vi "Steuerprogramm02-15.vi"() -> ()   [LabVIEW 2010]
uses:
  <vilib>/rvi/interface/nirviReadWriteControl/nirviReadWriteControl.xnode
  <vilib>/rvi/errors/niLvFpgaWhatHappensToTopLevelVI.ctl
  <vilib>/rvi/interface/common/niFpgaNodeNameForErrorReporting.ctl
  <vilib>/rvi/errors/niLvFpgaAdjustHostInterfaceError.vi
  gvbooleschRT.vi
  <vilib>/functionblocks/FB Core/FB Core.xnode
  <vilib>/functionblocks/Counter/Elapsed Timer/Elapsed Timer.vi
  <vilib>/functionblocks/NI_FunctionBlock Libraries.lvlib
  <vilib>/rvi/interface/nirviCloseFPGA/nirviCloseFPGA.xnode
  <vilib>/addons/control/pid/NI_PID_pid.lvlib
  C:/Users/HAGAR-IV/Desktop/Zeugs/Johnny/pertrasgc fpga/FPGA-Programm-10-14.vi
  C:/Users/HAGAR-IV/Desktop/Zeugs/markus/version feb 2012/FPGA Bitfiles/pertrasgcfpga2_FPGATarget_FPGA-Programm-10_16368CB6.lvbitx
  NiFpgaLv.dll
  <vilib>/Utility/error.llb/Error Cluster From Error Code.vi
  GVMWHorst.vi
  GVMethodenwechsel.vi
  GVHorstSP.vi
  GVZwangs.vi
  GVHK1Hz.vi
  GVHeizenLH.vi
  GVAIs.vi
  <vilib>/addons/control/pid/pid.llb/PID (DBL Array).vi
  GVTrapsMachs.vi
  GVaktuelleTDMS.vi
  GVECDs.vi
  GVZeitenZyklen.vi
  GVProbenvol.vi
  GVVentilposition.vi
  <vilib>/FPGAPlugInAG/cRIO-9114/niLvFpga_Close_cRIO-9114.vi
panel:
  in  "Methode speichern":bool
  in  "DetYMax":dbl
  in  "DetYMin":dbl
  in  "HK2YMax":dbl
  in  "HK2YMin":dbl
  in  "HK1YMax":dbl
  in  "HK1YMin":dbl
  out "ZyklusNummernGesamt":i32[](array[numeric])
  in  "Detektor":i32(ring) items=["ECD1", "ECD2"]
  out "Detektor":cluster{dbl[], dbl[]}[](graph)
  out "Zykluslängen [s]":dbl[](array[numeric])
  in  "veränderte Methode benutzen":bool
  in  "Methode verändern":bool
  in  "dargestellte Größe 2":i32(ring)=1 items=["T-MainCol3", "T-Trap1", "T-Trap2", "T-Stirling", "T-PreCol1", "T-PreCol2", "T-MainCol1", "T-MainCol2", "T-T-Line2", "T-MI1", "T-MI2", "T-MI3", "T-MI4", "T-MI5", "T-MI6", "F-MFM1", "T-MainCol4", "T-BHorst1", "T-BHorst2", "T-BHorst3", "T-BHorst4", "T-Oven1", "T-Oven2", "T-T-Line1", "F-MFM2", "P-Me-HP", "P-Me-LP", "P-Vac", "Ref-Turbo", "I-MS-AC", "I-Trap1", "I-Trap2", "Mod2/AI0", "Mod2/AI1", "Mod2/AI2", "Mod2/AI3", "Mod2/AI4", "Mod2/AI5", "Mod2/AI6", "Mod2/AI7", "Mod2/AI8", "Mod2/AI9", "Mod2/AI10", "Mod2/AI11", "Mod2/AI12", "Mod2/AI13", "Mod2/AI14", "Mod2/AI15", "Mod2/AI16", "Mod2/AI17", "Mod2/AI18", "Mod2/AI19", "Mod2/AI20", "Mod2/AI21", "Mod2/AI22", "Mod2/AI23", "Mod2/AI24", "Mod2/AI25", "Mod2/AI26", "Mod2/AI27", "Mod2/AI28", "Mod2/AI29", "Mod2/AI30", "Mod2/AI31", "Mod3/AI0", "Mod3/AI1", "Mod3/AI2", "Mod3/AI3", "Mod3/AI4", "Mod3/AI5", "Mod3/AI6", "Mod3/AI7", "Mod3/AI8", "Mod3/AI9", "Mod3/AI10", "Mod3/AI11", "Mod3/AI12", "Mod3/AI13", "Mod3/AI14", "Mod3/AI15", "Mod3/AI16", "Mod3/AI17", "Mod3/AI18", "Mod3/AI19", "Mod3/AI20", "Mod3/AI21", "Mod3/AI22", "Mod3/AI23", "Mod3/AI24", "Mod3/AI25", "Mod3/AI26", "Mod3/AI27", "Mod3/AI28", "Mod3/AI29", "Mod3/AI30", "Mod3/AI31", "U_Widr.Trap1 [V]", "Temp.Trap1 [°C]", "U_Widr.Trap2 [V]", "Temp.Trap2 [°C]", "Temp.Mach1 [°C]", "Temp.Mach2 [°C]", "MFC1B", "PressContr1A", "PressContr1B", "PressContr1C", "MFC1A", "PressContr1D", "MFC1A Integriert"]
  in  "Zeitachse2":i32(ring)=1 items=["Zykluszeit [s] Mod0", "Zykluszeit [s] Mod1", "Zykluszeit [s] Mod2A", "Zykluszeit [s] Mod2B"]
  out "Housekeeping2":cluster{dbl[], dbl[]}(graph)
  out "ZyklusNummern":i32[](array[numeric])
  in  "dargestellte Größe 1":i32(ring)=1 items=["T-MainCol3", "T-Trap1", "T-Trap2", "T-Stirling", "T-PreCol1", "T-PreCol2", "T-MainCol1", "T-MainCol2", "T-T-Line2", "T-MI1", "T-MI2", "T-MI3", "T-MI4", "T-MI5", "T-MI6", "F-MFM1", "T-MainCol4", "T-BHorst1", "T-BHorst2", "T-BHorst3", "T-BHorst4", "T-Oven1", "T-Oven2", "T-T-Line1", "F-MFM2", "P-Me-HP", "P-Me-LP", "P-Vac", "Ref-Turbo", "I-MS-AC", "I-Trap1", "I-Trap2", "Mod2/AI0", "Mod2/AI1", "Mod2/AI2", "Mod2/AI3", "Mod2/AI4", "Mod2/AI5", "Mod2/AI6", "Mod2/AI7", "Mod2/AI8", "Mod2/AI9", "Mod2/AI10", "Mod2/AI11", "Mod2/AI12", "Mod2/AI13", "Mod2/AI14", "Mod2/AI15", "Mod2/AI16", "Mod2/AI17", "Mod2/AI18", "Mod2/AI19", "Mod2/AI20", "Mod2/AI21", "Mod2/AI22", "Mod2/AI23", "Mod2/AI24", "Mod2/AI25", "Mod2/AI26", "Mod2/AI27", "Mod2/AI28", "Mod2/AI29", "Mod2/AI30", "Mod2/AI31", "Mod3/AI0", "Mod3/AI1", "Mod3/AI2", "Mod3/AI3", "Mod3/AI4", "Mod3/AI5", "Mod3/AI6", "Mod3/AI7", "Mod3/AI8", "Mod3/AI9", "Mod3/AI10", "Mod3/AI11", "Mod3/AI12", "Mod3/AI13", "Mod3/AI14", "Mod3/AI15", "Mod3/AI16", "Mod3/AI17", "Mod3/AI18", "Mod3/AI19", "Mod3/AI20", "Mod3/AI21", "Mod3/AI22", "Mod3/AI23", "Mod3/AI24", "Mod3/AI25", "Mod3/AI26", "Mod3/AI27", "Mod3/AI28", "Mod3/AI29", "Mod3/AI30", "Mod3/AI31", "U_Widr.Trap1 [V]", "Temp.Trap1 [°C]", "U_Widr.Trap2 [V]", "Temp.Trap2 [°C]", "Temp.Mach1 [°C]", "Temp.Mach2 [°C]", "MFC1B", "PressContr1A", "PressContr1B", "PressContr1C", "MFC1A", "PressContr1D", "MFC1A Integriert"]
  in  "Zeitachse1":i32(ring)=1 items=["Zykluszeit [s] Mod0", "Zykluszeit [s] Mod1", "Zykluszeit [s] Mod2A", "Zykluszeit [s] Mod2B"]
  out "Housekeeping1":cluster{dbl[], dbl[]}(graph)
  out "Big Ben, Methodenzeit, Zykluszeit0, Zykluszeit1, Zykluszeit2A, Zykluszeit2B":dbl[](array[numeric])
  in  "global stop RT":bool
  in  "Methode":i32(ring) items=["0"]
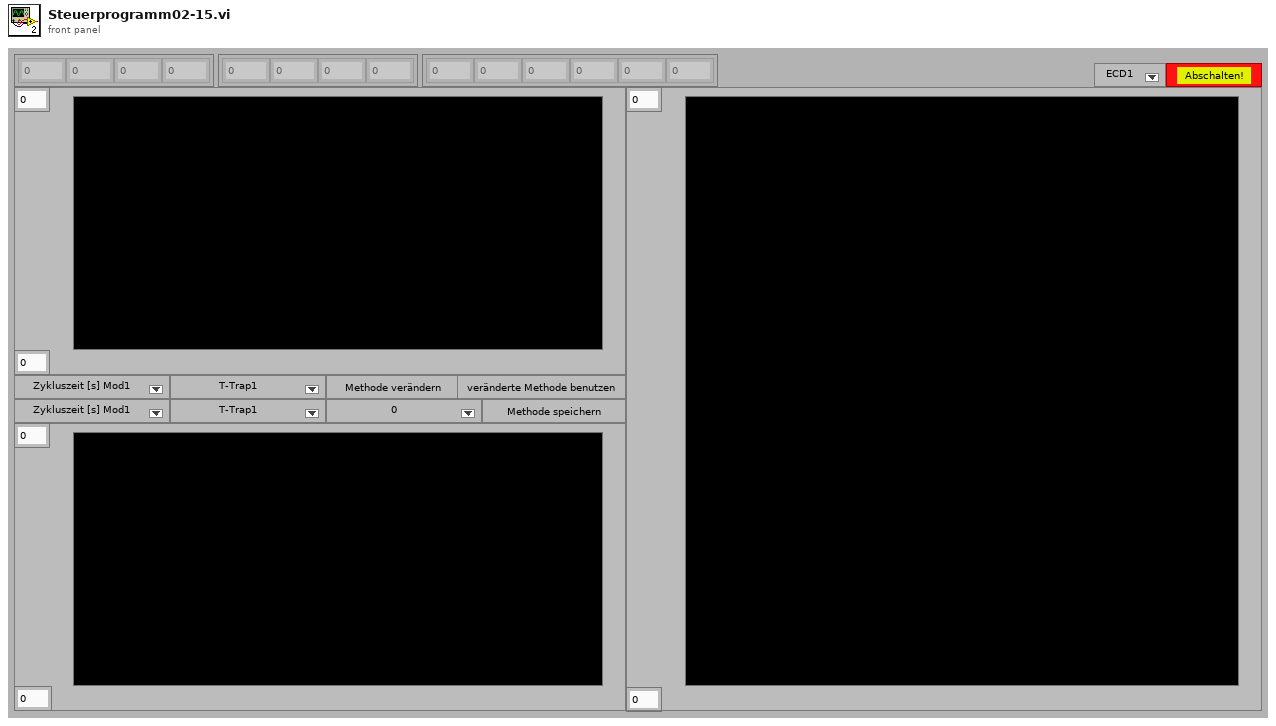
[diagram p1: front panel]
types:
  T1 = cluster{"Zykluslängen [s]":dbl[], "ZeitpktDIOsMod0":dbl[], "ZeitpktDIOsMod1":dbl[], "ZeitpktDIOsMod2A":dbl[], "ZeitpktDIOsMod2B":dbl[], "DIOsSPMod0":bool[][], "DIOsSPMod1":bool[][], "DIOsSPMod2A":bool[][], "DIOsSPMod2B":bool[][], "Mod0HorstZeitpkt":dbl[], "Mod1HorstZeitpkt":dbl[], "Mod2AHorstZeitpkt":dbl[], "Mod2BHorstZeitpkt":dbl[], "HorstSPMod0":dbl[][], "HorstSPMod1":dbl[][], "HorstSPMod2A":dbl[][], "HorstSPMod2B":dbl[][], "LangsameHeizungenSP":dbl[], "LHHeizen?":bool[], "ZPktFPGABoolesch":dbl[], "FPGABoolesch":bool[][], "ZeitpktFPGAPID":dbl[], "FPGAPID":cluster{"proportional gain (Kc)":fxp<+/-,16,8>, "integral gain (Kc*Ts/Ti)":fxp<+/-,16,8>, "derivative gain (Kc*Td/Ts)":fxp<+/-,16,8>}[][], "ZeitpktFPGAFixp":dbl[], "FPGAFixp":fxp<+/-,16,4>[][], "ZeitpktMach1":dbl[], "TempMach1":dbl[], "ZeitpktMach2":dbl[], "TempMach2":dbl[], "PIDs für \"träge\" Heizungen":cluster{"proportional gain (Kc)":dbl, "integral time (Ti, min)":dbl, "derivative time (Td, min)":dbl}[], "Zwangsbedingungen":dbl[][], "Dateien fürs MS schicken?":bool, "ZeitpunkteMPV":dbl[], "SPMPV":i32[], "ZeitpktMSa":dbl, "ZeitpktMSb":dbl, "Int.Start1":dbl, "Int.Stop1":dbl, "Int.Start2":dbl, "Int.Stop2":dbl, "Methodenname":string}[]
  T2 = cluster{"DIOsMod0Nr":i32[], "DIOsMod1Nr":i32[], "DIOsMod2ANr":i32[], "DIOsMod2BNr":i32[], "AIsLH":i32[], "Anzahl Horst/Modul":i32[], "Regler für den Probenfluß":i32, "StringSPvorgebenMod0":string[], "StringSPvorgebenMod1":string[], "StringSPvorgebenMod2A":string[], "StringSPvorgebenMod2B":string[], "StringMWAntwort0":string[], "StringMWAntwort1":string[], "StringMWAntwort2A":string[], "StringMWAntwort2B":string[], "UmrechnungHorst0":dbl[], "UmrechnungHorst1":dbl[], "UmrechnungHorst2A":dbl[], "UmrechnungHorst2B":dbl[], "StringMWabfragenMod0":string[], "StringMWabfragenMod1":string[], "StringMWabfragenMod2A":string[], "StringMWabfragenMod2B":string[], "Modul1/AI koeff":dbl[][], "Modul2/AI koeff":dbl[][], "Modul3/AI koeff":dbl[][], "Traps/MachsKoeff":dbl[][], "Modul1/AIsNamen":string[], "Modul2/AIsNamen":string[], "Modul3/AIsNamen":string[], "DIOsMod0Name":string[], "DIOsMod1Name":string[], "DIOsMod2AName":string[], "DIOsMod2BName":string[], "HorstMod0Name":string[], "HorstMod1Name":string[], "HorstMod2AName":string[], "HorstMod2BName":string[], "Startmethode":i32, "Dateiordner Housekeeping":path, "Dateiname Housekeeping":string, "DateiordnerECD1":path, "DateinameECD1":string, "DateiordnerECD2":path, "DateinameECD2":string, "NamenLangsameHeizungen":string[], "ModuleLH":i32[]}
  T3 = enum16{"open", "replace", "create", "open or create", "replace or create", "replace or create with confirmation"}
  T4 = cluster{"DIOsMod0Nr":i32[], "DIOsMod1Nr":i32[], "DIOsMod2ANr":i32[], "DIOsMod2BNr":i32[], "AIs für \"träge\" Heizungen":i32[], i32[], "AnschlüsseHorstMod0":enum8{"0", "1", "2", "3", "4", "5", "6", "7", "8"}[], "AnschlüsseHorstMod1":enum8{"0", "1", "2", "3", "4", "5", "6", "7", "8"}[], "AnschlüsseHorstMod2A":enum8{"0", "1", "2", "3", "4", "5", "6", "7", "8"}[], "AnschlüsseHorstMod2B":enum8{"0", "1", "2", "3", "4", "5", "6", "7", "8"}[], "StringSPvorgebenMod0":string[], "StringSPvorgebenMod1":string[], "StringSPvorgebenMod2A":string[], "StringSPvorgebenMod2B":string[], "StringMWAntwort0":string[], "StringMWAntwort1":string[], "StringMWAntwort2A":string[], "StringMWAntwort2B":string[], "UmrechnungHorst0":dbl[], "UmrechnungHorst1":dbl[], "UmrechnungHorst2A":dbl[], "UmrechnungHorst2B":dbl[], "StringMWabfragenMod0":string[], "StringMWabfragenMod1":string[], "StringMWabfragenMod2A":string[], "StringMWabfragenMod2B":string[], "Modul1/AI koeff":dbl[][], "Modul2/AI koeff":dbl[][], "Modul3/AI koeff":dbl[][], "Traps/MachKoeff":dbl[][], "AIsNamen":string[], "DIOsMod0Name":string[], "DIOsMod1Name":string[], "DIOsMod2AName":string[], "DIOsMod2BName":string[], "HorstMod0Name":string[], "HorstMod1Name":string[], "HorstMod2AName":string[], "HorstMod2BName":string[], "Startmethode":i32, "Dateiordner Housekeeping":path, "Dateiname Housekeeping":string, "DateiordnerECD1":path, "DateinameECD1":string, "DateiordnerECD2":path, "DateinameECD2":string}
  T5 = cluster{"Zykluslängen [s]":dbl[], "ZeitpktDIOsMod0":dbl[], "ZeitpktDIOsMod1":dbl[], "ZeitpktDIOsMod2A":dbl[], "ZeitpktDIOsMod2B":dbl[], "DIOsSPMod0":bool[][], "DIOsSPMod1":bool[][], "DIOsSPMod2A":bool[][], "DIOsSPMod2B":bool[][], "Mod0HorstZeitpkt":dbl[], "Mod1HorstZeitpkt":dbl[], "Mod2AHorstZeitpkt":dbl[], "Mod2BHorstZeitpkt":dbl[], "HorstSPMod0":dbl[][], "HorstSPMod1":dbl[][], "HorstSPMod2A":dbl[][], "HorstSPMod2B":dbl[][], "LangsameHeizungenSP":dbl[], "LHHeizen?":bool[], "ZPktFPGABoolesch":dbl[], "FPGABoolesch":bool[][], "ZeitpktFPGAPID":dbl[], "FPGAPID":cluster{"proportional gain (Kc)":fxp<+/-,16,8>, "integral gain (Kc*Ts/Ti)":fxp<+/-,16,8>, "derivative gain (Kc*Td/Ts)":fxp<+/-,16,8>}[][], "ZeitpktFPGAFixp":dbl[], "FPGAFixp":fxp<+/-,16,4>[][], "ZeitpktMach1":dbl[], "TempMach1":dbl[], "ZeitpktMach2":dbl[], "TempMach2":dbl[], "PIDs für \"träge\" Heizungen":cluster{"proportional gain (Kc)":dbl, "integral time (Ti, min)":dbl, "derivative time (Td, min)":dbl}[], "Zwangsbedingungen":dbl[][], "Text0 MS-Datei":string, "Info":string, "wie wird gespeichert?":u16, "Speicherlänge":string, "Dateien fürs MS schicken?":bool, "Pfad MS-Datei CRIO":path}[]
  T6 = cluster{"DIOsMod0Nr":i32[], "DIOsMod1Nr":i32[], "DIOsMod2ANr":i32[], "DIOsMod2BNr":i32[], "AIs für \"träge\" Heizungen":i32[], i32[], "AnschlüsseHorstMod0":enum8{"0", "1", "2", "3", "4", "5", "6", "7", "8"}[], "AnschlüsseHorstMod1":enum8{"0", "1", "2", "3", "4", "5", "6", "7", "8"}[], "AnschlüsseHorstMod2A":enum8{"0", "1", "2", "3", "4", "5", "6", "7", "8"}[], "AnschlüsseHorstMod2B":enum8{"0", "1", "2", "3", "4", "5", "6", "7", "8"}[], "StringSPvorgebenMod0":string[], "StringSPvorgebenMod1":string[], "StringSPvorgebenMod2A":string[], "StringSPvorgebenMod2B":string[], "StringMWAntwort0":string[], "StringMWAntwort1":string[], "StringMWAntwort2A":string[], "StringMWAntwort2B":string[], "UmrechnungHorst0":dbl[], "UmrechnungHorst1":dbl[], "UmrechnungHorst2A":dbl[], "UmrechnungHorst2B":dbl[], "StringMWabfragenMod0":string[], "StringMWabfragenMod1":string[], "StringMWabfragenMod2A":string[], "StringMWabfragenMod2B":string[], "Modul1/AI koeff":dbl[][], "Modul2/AI koeff":dbl[][], "Modul3/AI koeff":dbl[][], "Traps/MachKoeff":dbl[][], "AIsNamen":string[], "DIOsMod0Name":string[], "DIOsMod1Name":string[], "DIOsMod2AName":string[], "DIOsMod2BName":string[], "HorstMod0Name":string[], "HorstMod1Name":string[], "HorstMod2AName":string[], "HorstMod2BName":string[], "Startmethode":i32, "Dateiordner Housekeeping":path, "Dateiname Housekeeping":string}
  T7 = cluster{"Zyklus1":i32, "Zeitachse1":i32, "dargestellte Größe 1":i32, "Zyklus2":i32, "Zeitachse2":i32, "dargestellte Größe 2":i32}
  T8 = typedef "niFpgaNodeNameForErrorReporting.ctl" = enum16{"Open FPGA VI Reference", "Read/Write Control", "Invoke Method: Abort", "Invoke Method: Acknowledge IRQ", "Invoke Method: Download", "Invoke Method: FIFO.Configure", "Invoke Method: FIFO.Read", "Invoke Method: FIFO.Start", "Invoke Method: FIFO.Stop", "Invoke Method: FIFO.Write", "Invoke Method: Reset", "Invoke Method: Run", "Invoke Method: Wait on IRQ", "Close FPGA VI Reference"}
  T9 = typedef "niLvFpgaWhatHappensToTopLevelVI.ctl" = enum16{"top level VI scripted behind XNode", "top level VI inlined behind XNode"}
  T10 = cluster{"DIOsMod0Name":string[], "DIOsMod1Name":string[], "DIOsMod2AName":string[], "DIOsMod2BName":string[], "HorstMod0Name":string[], "HorstMod1Name":string[], "HorstMod2AName":string[], "HorstMod2BName":string[], "NamenLangsameHeizungen":string[]}
  T11 = cluster{"Dateiordner Housekeeping":path, "DateiordnerECD1":path, "DateiordnerECD2":path, "Dateiname Housekeeping":string, "DateinameECD1":string, "DateinameECD2":string, "tdms0":refnum<k34>, "tdms1":refnum<k34>, "tdms0":refnum<k34>, "tdms1":refnum<k34>, "tdms0":refnum<k34>, "tdms1":refnum<k34>}
  T12 = cluster{"Zykluslängen [s]":dbl[], "ZeitpktDIOsMod0":dbl[], "ZeitpktDIOsMod1":dbl[], "ZeitpktDIOsMod2A":dbl[], "ZeitpktDIOsMod2B":dbl[], "DIOsSPMod0":bool[][], "DIOsSPMod1":bool[][], "DIOsSPMod2A":bool[][], "DIOsSPMod2B":bool[][], "Mod0HorstZeitpkt":dbl[], "Mod1HorstZeitpkt":dbl[], "Mod2AHorstZeitpkt":dbl[], "Mod2BHorstZeitpkt":dbl[], "HorstSPMod0":dbl[][], "HorstSPMod1":dbl[][], "HorstSPMod2A":dbl[][], "HorstSPMod2B":dbl[][], "LangsameHeizungenSP":dbl[], "LHHeizen?":bool[], "ZPktFPGABoolesch":dbl[], "FPGABoolesch":bool[][], "ZeitpktFPGAPID":dbl[], "FPGAPID":cluster{"proportional gain (Kc)":fxp<+/-,16,8>, "integral gain (Kc*Ts/Ti)":fxp<+/-,16,8>, "derivative gain (Kc*Td/Ts)":fxp<+/-,16,8>}[][], "ZeitpktFPGAFixp":dbl[], "FPGAFixp":fxp<+/-,16,4>[][], "ZeitpktMach1":dbl[], "TempMach1":dbl[], "ZeitpktMach2":dbl[], "TempMach2":dbl[], "PIDs für \"träge\" Heizungen":cluster{"proportional gain (Kc)":dbl, "integral time (Ti, min)":dbl, "derivative time (Td, min)":dbl}[], "Zwangsbedingungen":dbl[][], "Dateien fürs MS schicken?":bool, "ZeitpunkteMPV":dbl[], "SPMPV":i32[], "ZeitpktMSa":dbl, "ZeitpktMSb":dbl, "Int.Start1":dbl, "Int.Stop1":dbl, "Int.Start2":dbl, "Int.Stop2":dbl, "Methodenname":string}
  T13 = cluster{"proportional gain (Kc)":fxp<+/-,16,8>, "integral gain (Kc*Ts/Ti)":fxp<+/-,16,8>, "derivative gain (Kc*Td/Ts)":fxp<+/-,16,8>}[][]
  T14 = cluster{"proportional gain (Kc)":dbl, "integral time (Ti, min)":dbl, "derivative time (Td, min)":dbl}[]
  T15 = cluster{"Heizen?LH[0]":bool, "Heizen?LH[1]":bool, "Heizen?LH[2]":bool, "Heizen?LH[3]":bool, "Heizen?LH[4]":bool, "Heizen?LH[5]":bool}
  T16 = cluster{"[0]":u32, "[1]":u32, "[2]":u32, "[3]":u32, "[4]":u32, "[5]":u32}
  T17 = cluster{cluster{"ZeitpktDIOsMod2B":dbl[]}[], cluster{"DIOsSPMod2B":bool[][]}[], cluster{"Mod2BHorstZeitpkt":dbl[]}[], cluster{"HorstSPMod2B":dbl[][]}[], "LHHeizen?":bool[], "ZPktFPGABoolesch":dbl[], "FPGABoolesch":bool[][], "ZeitpktFPGAPID":dbl[], "FPGAPID":cluster{"proportional gain (Kc)":fxp<+/-,16,8>, "integral gain (Kc*Ts/Ti)":fxp<+/-,16,8>, "derivative gain (Kc*Td/Ts)":fxp<+/-,16,8>}[][], "ZeitpktFPGAFixp":dbl[], "FPGAFixp":fxp<+/-,16,4>[][], "ZeitpktMach1":dbl[], "TempMach1":dbl[], "ZeitpktMach2":dbl[], "TempMach2":dbl[], "ZeitpunkteMPV":dbl[], "SPMPV":i32[]}
  T18 = cluster{"ZyklusNummern":i32[], "ZeilennummernDIOs":i32[], "ZwangsDIO?":cluster{bool[]}[], "ZeilennummernHorst":i32[], "ZwangsHorst?":cluster{bool[]}[], "ZeileFPGABoolesch":i32, "ZwangsFPGABoolesch?":bool[], "ZeileFPGAPID":i32, "ZeileFPGAFixp":i32, "ZeileMach1":i32, "ZeileMach2":i32, "ZeilennummerMPV":i32}
  T19 = cluster{"Zyklusnummern 0, 1, 2A, 2B":i32[], i32[], "ZwangsDIO?":cluster{bool[]}[], i32[], "ZwangsHorst?":cluster{bool[]}[], i32, "ZwangsFPGABoolesch?":bool[], i32, i32, i32, i32, "ZeilennummerMPV":i32}
  T20 = cluster{string[], string[], string[], dbl[], dbl[], dbl[]}
  T21 = cluster{string[], string[], string[], string, string}
  T22 = cluster{"Befehle1":string[], "Befehle2":string[], "Befehle3":string[]}
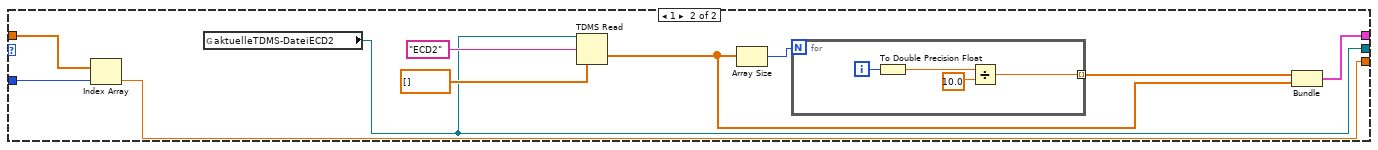
[diagram p6: hidden frame]
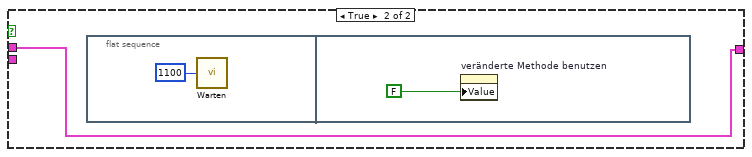
[diagram p7: hidden frame]
diagram:
  (unwired) T4 {"DIOsMod0Nr"=[], "DIOsMod1Nr"=[], "DIOsMod2ANr"=[], "DIOsMod2BNr"=[], "AIs für \"träge\" Heizungen"=[], [], "AnschlüsseHorstMod0"=[], "AnschlüsseHorstMod1"=[], "AnschlüsseHorstMod2A"=[], "AnschlüsseHorstMod2B"=[], "StringSPvorgebenMod0"=[], "StringSPvorgebenMod1"=[], "StringSPvorgebenMod2A"=[], "StringSPvorgebenMod2B"=[], "StringMWAntwort0"=[], "StringMWAntwort1"=[], "StringMWAntwort2A"=[], "StringMWAntwort2B"=[], "UmrechnungHorst0"=[], "UmrechnungHorst1"=[], "UmrechnungHorst2A"=[], "UmrechnungHorst2B"=[], "StringMWabfragenMod0"=[], "StringMWabfragenMod1"=[], "StringMWabfragenMod2A"=[], "StringMWabfragenMod2B"=[], "Modul1/AI koeff"=[], "Modul2/AI koeff"=[], "Modul3/AI koeff"=[], "Traps/MachKoeff"=[], "AIsNamen"=[], "DIOsMod0Name"=[], "DIOsMod1Name"=[], "DIOsMod2AName"=[], "DIOsMod2BName"=[], "HorstMod0Name"=[], "HorstMod1Name"=[], "HorstMod2AName"=[], "HorstMod2BName"=[], "Startmethode"=0, "Dateiordner Housekeeping"=path "", "Dateiname Housekeeping"="", "DateiordnerECD1"=path "", "DateinameECD1"="", "DateiordnerECD2"=path "", "DateinameECD2"=""} ("Einstellungen")
  (unwired) T5 [{"Zykluslängen [s]"=[180.0, 180.0, 180.0, 180.0], "ZeitpktDIOsMod0"=[0.0, 180.0], "ZeitpktDIOsMod1"=[0.0, 2.0, 15.0, 60.0, 61.0, 70.0, 80.0, 170.0, 180.0], "ZeitpktDIOsMod2A"=[0.0, 180.0], "ZeitpktDIOsMod2B"=[0.0, 60.0, 180.0], "DIOsSPMod0"=[[FALSE], [FALSE]], "DIOsSPMod1"=[[TRUE, TRUE, FALSE, TRUE, FALSE, TRUE, TRUE, TRUE, FALSE, FALSE, TRUE, FALSE, FALSE, FALSE, FALSE, FALSE, FALSE, TRUE], [TRUE, FALSE, FALSE, TRUE, FALSE, TRUE, TRUE, TRUE, FALSE, FALSE, TRUE, FALSE, FALSE, FALSE, FALSE, FALSE, FALSE, TRUE], [TRUE, FALSE, FALSE, FALSE, FALSE, TRUE, TRUE, FALSE, FALSE, FALSE, TRUE, FALSE, FALSE, FALSE, FALSE, FALSE, TRUE, TRUE], [TRUE, FALSE, FALSE, FALSE, FALSE, FALSE, TRUE, FALSE, FALSE, FALSE, TRUE, FALSE, FALSE, FALSE, FALSE, FALSE, TRUE, TRUE], [TRUE, FALSE, FALSE, FALSE, FALSE, FALSE, TRUE, FALSE, FALSE, FALSE, TRUE, FALSE, FALSE, FALSE, FALSE, FALSE, TRUE, TRUE], [TRUE, FALSE, FALSE, FALSE, FALSE, FALSE, TRUE, FALSE, FALSE, FALSE, TRUE, FALSE, FALSE, FALSE, FALSE, FALSE, TRUE, TRUE], [TRUE, FALSE, FALSE, FALSE, FALSE, FALSE, TRUE, FALSE, FALSE, FALSE, TRUE, FALSE, FALSE, FALSE, FALSE, FALSE, FALSE, TRUE], [TRUE, FALSE, FALSE, FALSE, FALSE, FALSE, TRUE, FALSE, FALSE, FALSE, TRUE, FALSE, FALSE, FALSE, FALSE, FALSE, FALSE, TRUE], [TRUE, FALSE, FALSE, FALSE, FALSE, FALSE, TRUE, FALSE, FALSE, FALSE, TRUE, FALSE, FALSE, FALSE, FALSE, FALSE, FALSE, TRUE]], "DIOsSPMod2A"=[[FALSE], [FALSE]], "DIOsSPMod2B"=[[FALSE], [FALSE]], "Mod0HorstZeitpkt"=[0.0, 180.0], "Mod1HorstZeitpkt"=[0.0, 55.0, 75.0, 180.0], "Mod2AHorstZeitpkt"=[0.0, 20.0, 180.0], "Mod2BHorstZeitpkt"=[0.0, 380.0], "HorstSPMod0"=[[2.66], [2.66]], "HorstSPMod1"=[[1.9, 0.0, 1.2], [0.0, 0.0, 1.2], [1.9, 0.0, 1.2], [1.9, 0.0, 1.2]], "HorstSPMod2A"=[[300.0], [300.0], [300.0]], "HorstSPMod2B"=[[0.0], [0.0]], "LangsameHeizungenSP"=[60.0, 220.0, 120.0, 60.0, 110.0, 0.0], "LHHeizen?"=[FALSE, TRUE, TRUE, FALSE, TRUE, FALSE], "ZPktFPGABoolesch"=[0.0, 60.0, 75.0, 180.0], "FPGABoolesch"=[[FALSE, FALSE, FALSE, FALSE, TRUE, FALSE], [FALSE, FALSE, TRUE, FALSE, TRUE, FALSE], [FALSE, FALSE, FALSE, FALSE, TRUE, FALSE], [FALSE, FALSE, FALSE, FALSE, TRUE, FALSE]], "ZeitpktFPGAPID"=[0.0, 60.0, 180.0], "FPGAPID"=[[{"proportional gain (Kc)"=5.0, "integral gain (Kc*Ts/Ti)"=0.0, "derivative gain (Kc*Td/Ts)"=0.0}, {"proportional gain (Kc)"=1.0, "integral gain (Kc*Ts/Ti)"=1.66796875, "derivative gain (Kc*Td/Ts)"=0.0}, {"proportional gain (Kc)"=5.0, "integral gain (Kc*Ts/Ti)"=0.03515625, "derivative gain (Kc*Td/Ts)"=0.0234375}, {"proportional gain (Kc)"=1.0, "integral gain (Kc*Ts/Ti)"=1.66796875, "derivative gain (Kc*Td/Ts)"=0.0}], [{"proportional gain (Kc)"=5.0, "integral gain (Kc*Ts/Ti)"=0.0, "derivative gain (Kc*Td/Ts)"=0.0}, {"proportional gain (Kc)"=1.0, "integral gain (Kc*Ts/Ti)"=1.66796875, "derivative gain (Kc*Td/Ts)"=0.0}, {"proportional gain (Kc)"=5.0, "integral gain (Kc*Ts/Ti)"=0.03515625, "derivative gain (Kc*Td/Ts)"=0.0234375}, {"proportional gain (Kc)"=1.0, "integral gain (Kc*Ts/Ti)"=1.66796875, "derivative gain (Kc*Td/Ts)"=0.0}], [{"proportional gain (Kc)"=0.0, "integral gain (Kc*Ts/Ti)"=0.0, "derivative gain (Kc*Td/Ts)"=0.0}, {"proportional gain (Kc)"=0.0, "integral gain (Kc*Ts/Ti)"=0.0, "derivative gain (Kc*Td/Ts)"=0.0}, {"proportional gain (Kc)"=2.0, "integral gain (Kc*Ts/Ti)"=0.03125, "derivative gain (Kc*Td/Ts)"=0.01953125}, {"proportional gain (Kc)"=0.0, "integral gain (Kc*Ts/Ti)"=0.0, "derivative gain (Kc*Td/Ts)"=0.0}], [{"proportional gain (Kc)"=0.0, "integral gain (Kc*Ts/Ti)"=0.0, "derivative gain (Kc*Td/Ts)"=0.0}, {"proportional gain (Kc)"=0.0, "integral gain (Kc*Ts/Ti)"=0.0, "derivative gain (Kc*Td/Ts)"=0.0}, {"proportional gain (Kc)"=2.0, "integral gain (Kc*Ts/Ti)"=0.03125, "derivative gain (Kc*Td/Ts)"=0.01953125}, {"proportional gain (Kc)"=0.0, "integral gain (Kc*Ts/Ti)"=0.0, "derivative gain (Kc*Td/Ts)"=0.0}], [{"proportional gain (Kc)"=0.0, "integral gain (Kc*Ts/Ti)"=0.0, "derivative gain (Kc*Td/Ts)"=0.0}, {"proportional gain (Kc)"=0.0, "integral gain (Kc*Ts/Ti)"=0.0, "derivative gain (Kc*Td/Ts)"=0.0}, {"proportional gain (Kc)"=2.0, "integral gain (Kc*Ts/Ti)"=0.03125, "derivative gain (Kc*Td/Ts)"=0.01953125}, {"proportional gain (Kc)"=0.0, "integral gain (Kc*Ts/Ti)"=0.0, "derivative gain (Kc*Td/Ts)"=0.0}]], "ZeitpktFPGAFixp"=[0.0, 60.0, 75.0, 180.0], "FPGAFixp"=[[0.0, 0.0, 0.0, 0.0, 0.0, 0.0, 2.85009765625, 0.0], [4.59423828125, 4.599365234375, 1.699951171875, 0.0, 0.0, 0.0, 2.85009765625, 0.0], [0.0, 0.0, 0.0, 0.0, 0.0, 0.0, 2.85009765625, 0.0], [0.0, 0.0, 0.0, 0.0, 0.0, 0.0, 2.85009765625, 0.0]], "ZeitpktMach1"=[0.0, 1.0, 100.0, 101.0, 177.0, 178.0, 180.0], "TempMach1"=[50.0, 50.0, 50.0, 250.0, 250.0, 50.0, 50.0], "ZeitpktMach2"=[0.0, 0.0, 120.0], "TempMach2"=[0.0, 0.0, 0.0], "PIDs für \"träge\" Heizungen"=[{"proportional gain (Kc)"=1.0, "integral time (Ti, min)"=0.01, "derivative time (Td, min)"=0.0}, {"proportional gain (Kc)"=2.0, "integral time (Ti, min)"=1.0, "derivative time (Td, min)"=0.0}, {"proportional gain (Kc)"=4.0, "integral time (Ti, min)"=1.0, "derivative time (Td, min)"=0.0}, {"proportional gain (Kc)"=1.0, "integral time (Ti, min)"=0.01, "derivative time (Td, min)"=0.0}, {"proportional gain (Kc)"=2.0, "integral time (Ti, min)"=0.0, "derivative time (Td, min)"=0.0}, {"proportional gain (Kc)"=1.0, "integral time (Ti, min)"=0.01, "derivative time (Td, min)"=0.0}], "Zwangsbedingungen"=[[3.0, 4.0, 100.0, 23.0, 4.0, 200.0, 0.0, 0.0]], "Text0 MS-Datei"="text0", "Info"="info", "wie wird gespeichert?"=0, "Speicherlänge"="100", "Dateien fürs MS schicken?"=FALSE, "Pfad MS-Datei CRIO"=path "c:/"}] ("Eingang 2")
  (unwired) T6 {"DIOsMod0Nr"=[32], "DIOsMod1Nr"=[5, 6, 7, 10, 11, 14, 15, 16, 17, 18, 20, 23, 25, 26, 27, 28, 29, 30], "DIOsMod2ANr"=[33], "DIOsMod2BNr"=[34], "AIs für \"träge\" Heizungen"=[17, 6, 0, 19, 21, 23], [1, 3, 1, 1], "AnschlüsseHorstMod0"=[enum."1"], "AnschlüsseHorstMod1"=[enum."1", enum."1", enum."1"], "AnschlüsseHorstMod2A"=[enum."1"], "AnschlüsseHorstMod2B"=[enum."1"], "StringSPvorgebenMod0"=[":060A020121"], "StringSPvorgebenMod1"=[":060B020121", ":0618020121", ":060D020121"], "StringSPvorgebenMod2A"=[":0519010104"], "StringSPvorgebenMod2B"=[":060C020121 "], "StringMWAntwort0"=[":060A020121"], "StringMWAntwort1"=[":060B020121", ":0618020121", ":060D020121"], "StringMWAntwort2A"=[":0619020121"], "StringMWAntwort2B"=[":060C020121"], "UmrechnungHorst0"=[0.0003125], "UmrechnungHorst1"=[9.375e-05, 9.375e-05, 9.375e-05], "UmrechnungHorst2A"=[1.0], "UmrechnungHorst2B"=[9.375e-05], "StringMWabfragenMod0"=[":060A0401210120"], "StringMWabfragenMod1"=[":060B0401210120", ":06180401210120", ":060D0401210120"], "StringMWabfragenMod2A"=[":06190401210120"], "StringMWabfragenMod2B"=[":060C0401210120"], "Modul1/AI koeff"=[[-249.333, 111.873, 2.1471], [-249.333, 111.873, 2.1471], [-249.333, 111.873, 2.1471], [-249.333, 111.873, 2.1471], [-237.2852, -153.162, 6.0782], [-237.2852, -153.162, 6.0782], [-249.333, 111.873, 2.1471], [-249.333, 111.873, 2.1471], [-249.333, 111.873, 2.1471], [-249.333, 111.873, 2.1471], [-249.333, 111.873, 2.1471], [-249.333, 111.873, 2.1471], [-249.333, 111.873, 2.1471], [-249.333, 111.873, 2.1471], [-249.333, 111.873, 2.1471], [0.0, 1.0, 0.0], [-249.333, 111.873, 2.1471], [-249.333, 111.873, 2.1471], [-249.333, 111.873, 2.1471], [-249.333, 111.873, 2.1471], [-249.333, 111.873, 2.1471], [-249.333, 111.873, 2.1471], [-249.333, 111.873, 2.1471], [-249.333, 111.873, 2.1471], [0.0, 1.0, 0.0], [0.0, 1.0, 0.0], [0.0, 1.0, 0.0], [0.0, 1.0, 0.0], [0.0, 1.0, 0.0], [0.0, 1.0, 0.0], [0.0, 1.0, 0.0], [0.0, 1.0, 0.0]], "Modul2/AI koeff"=[[0.0, 1.0, 0.0], [0.0, 1.0, 0.0], [0.0, 1.0, 0.0], [0.0, 1.0, 0.0], [0.0, 1.0, 0.0], [0.0, 1.0, 0.0], [0.0, 1.0, 0.0], [0.0, 1.0, 0.0], [0.0, 1.0, 0.0], [0.0, 1.0, 0.0], [0.0, 1.0, 0.0], [0.0, 1.0, 0.0], [0.0, 1.0, 0.0], [0.0, 1.0, 0.0], [0.0, 1.0, 0.0], [0.0, 1.0, 0.0], [0.0, 1.0, 0.0], [0.0, 1.0, 0.0], [0.0, 1.0, 0.0], [0.0, 1.0, 0.0], [0.0, 1.0, 0.0], [0.0, 1.0, 0.0], [0.0, 1.0, 0.0], [0.0, 1.0, 0.0], [0.0, 1.0, 0.0], [0.0, 1.0, 0.0], [0.0, 1.0, 0.0], [0.0, 1.0, 0.0], [0.0, 1.0, 0.0], [0.0, 1.0, 0.0], [0.0, 1.0, 0.0], [0.0, 1.0, 0.0]], "Modul3/AI koeff"=[[0.0, 1.0, 0.0], [0.0, 1.0, 0.0], [0.0, 1.0, 0.0], [0.0, 1.0, 0.0], [0.0, 1.0, 0.0], [0.0, 1.0, 0.0], [0.0, 1.0, 0.0], [0.0, 1.0, 0.0], [0.0, 1.0, 0.0], [0.0, 1.0, 0.0], [0.0, 1.0, 0.0], [0.0, 1.0, 0.0], [0.0, 1.0, 0.0], [0.0, 1.0, 0.0], [0.0, 1.0, 0.0], [0.0, 1.0, 0.0], [0.0, 1.0, 0.0], [0.0, 1.0, 0.0], [0.0, 1.0, 0.0], [0.0, 1.0, 0.0], [0.0, 1.0, 0.0], [0.0, 1.0, 0.0], [0.0, 1.0, 0.0], [0.0, 1.0, 0.0], [0.0, 1.0, 0.0], [0.0, 1.0, 0.0], [0.0, 1.0, 0.0], [0.0, 1.0, 0.0], [0.0, 1.0, 0.0], [0.0, 1.0, 0.0], [0.0, 1.0, 0.0], [0.0, 1.0, 0.0]], "Traps/MachKoeff"=[[0.0, 1.0, 0.0], [-249.333, 111.873, 2.1471], [0.0, 1.0, 0.0], [-249.333, 111.873, 2.1471], [-237.2852, 153.1621, 6.0782], [-237.2852, 153.1621, 6.0782]], "AIsNamen"=["T-MainCol3", "T-Trap1", "T-Trap2", "T-Stirling", "T-PreCol1", "T-PreCol2", "T-MainCol1", "T-MainCol2", "T-T-Line2", "T-MI1", "T-MI2", "T-MI3", "T-MI4", "T-MI5", "T-MI6", "F-MFM1", "T-MainCol4", "T-BHorst1", "T-BHorst2", "T-BHorst3", "T-BHorst4", "T-Oven1", "T-Oven2", "T-T-Line1", "F-MFM2", "P-Me-HP", "P-Me-LP", "P-Vac", "Ref-Turbo", "I-MS-AC", "I-Trap1", "I-Trap2", "Mod2/AI0", "Mod2/AI1", "Mod2/AI2", "Mod2/AI3", "Mod2/AI4", "Mod2/AI5", "Mod2/AI6", "Mod2/AI7", "Mod2/AI8", "Mod2/AI9", "Mod2/AI10", "Mod2/AI11", "Mod2/AI12", "Mod2/AI13", "Mod2/AI14", "Mod2/AI15", "Mod2/AI16", "Mod2/AI17", "Mod2/AI18", "Mod2/AI19", "Mod2/AI20", "Mod2/AI21", "Mod2/AI22", "Mod2/AI23", "Mod2/AI24", "Mod2/AI25", "Mod2/AI26", "Mod2/AI27", "Mod2/AI28", "Mod2/AI29", "Mod2/AI30", "Mod2/AI31", "Mod3/AI0", "Mod3/AI1", "Mod3/AI2", "Mod3/AI3", "Mod3/AI4", "Mod3/AI5", "Mod3/AI6", "Mod3/AI7", "Mod3/AI8", "Mod3/AI9", "Mod3/AI10", "Mod3/AI11", "Mod3/AI12", "Mod3/AI13", "Mod3/AI14", "Mod3/AI15", "Mod3/AI16", "Mod3/AI17", "Mod3/AI18", "Mod3/AI19", "Mod3/AI20", "Mod3/AI21", "Mod3/AI22", "Mod3/AI23", "Mod3/AI24", "Mod3/AI25", "Mod3/AI26", "Mod3/AI27", "Mod3/AI28", "Mod3/AI29", "Mod3/AI30", "Mod3/AI31"], "DIOsMod0Name"=["blindDIO0"], "DIOsMod1Name"=["on/off P-MS", "MS Start", "MS Stop", "FanMach1", "FanReserve", "Valve1A", "on/off PrePump", "Air-In", "on/off VacP2", "on/off VacP1", "S1D", "FanMach2", "S1C", "on/off Stirling", "S1B", "S1A", "Valve1B", "on/off Turbo"], "DIOsMod2AName"=["blindDIO2A"], "DIOsMod2BName"=["blindDIO2B"], "HorstMod0Name"=["MFC1B"], "HorstMod1Name"=["PressContr1A", "PressContr1B", "PressContr1C"], "HorstMod2AName"=["MFC1A"], "HorstMod2BName"=["PressContr1D"], "Startmethode"=0, "Dateiordner Housekeeping"=path "C:/data", "Dateiname Housekeeping"="test"} ("Einstellungen")
  (unwired) T6 {"DIOsMod0Nr"=[32], "DIOsMod1Nr"=[5, 6, 7, 10, 11, 14, 15, 16, 17, 18, 20, 23, 25, 26, 27, 28, 29, 30], "DIOsMod2ANr"=[33], "DIOsMod2BNr"=[34], "AIs für \"träge\" Heizungen"=[17, 6, 0, 19, 21, 23], [1, 3, 1, 1], "AnschlüsseHorstMod0"=[enum."1"], "AnschlüsseHorstMod1"=[enum."1", enum."1", enum."1"], "AnschlüsseHorstMod2A"=[enum."1"], "AnschlüsseHorstMod2B"=[enum."1"], "StringSPvorgebenMod0"=[":060A020121"], "StringSPvorgebenMod1"=[":060B020121", ":0618020121", ":060D020121"], "StringSPvorgebenMod2A"=[":0619020121"], "StringSPvorgebenMod2B"=[":060C020121"], "StringMWAntwort0"=[":060A020121"], "StringMWAntwort1"=[":060B020121", ":0618020121", ":060D020121"], "StringMWAntwort2A"=[":0619020121"], "StringMWAntwort2B"=[":060C020121"], "UmrechnungHorst0"=[0.0003125], "UmrechnungHorst1"=[9.375e-05, 9.375e-05, 9.375e-05], "UmrechnungHorst2A"=[0.046875], "UmrechnungHorst2B"=[9.375e-05], "StringMWabfragenMod0"=[":060A0401210120"], "StringMWabfragenMod1"=[":060B0401210120", ":06180401210120", ":060D0401210120"], "StringMWabfragenMod2A"=[":06190401210120"], "StringMWabfragenMod2B"=[":060C0401210120"], "Modul1/AI koeff"=[[-249.333, 111.873, 2.1471], [-249.333, 111.873, 2.1471], [-249.333, 111.873, 2.1471], [-249.333, 111.873, 2.1471], [-237.2852, -153.162, 6.0782], [-237.2852, -153.162, 6.0782], [-249.333, 111.873, 2.1471], [-249.333, 111.873, 2.1471], [-249.333, 111.873, 2.1471], [-249.333, 111.873, 2.1471], [-249.333, 111.873, 2.1471], [-249.333, 111.873, 2.1471], [-249.333, 111.873, 2.1471], [-249.333, 111.873, 2.1471], [-249.333, 111.873, 2.1471], [0.0, 1.0, 0.0], [-249.333, 111.873, 2.1471], [-249.333, 111.873, 2.1471], [-249.333, 111.873, 2.1471], [-249.333, 111.873, 2.1471], [-249.333, 111.873, 2.1471], [-249.333, 111.873, 2.1471], [-249.333, 111.873, 2.1471], [-249.333, 111.873, 2.1471], [0.0, 1.0, 0.0], [0.0, 1.0, 0.0], [0.0, 1.0, 0.0], [0.0, 1.0, 0.0], [0.0, 1.0, 0.0], [0.0, 1.0, 0.0], [0.0, 1.0, 0.0], [0.0, 1.0, 0.0]], "Modul2/AI koeff"=[[0.0, 1.0, 0.0], [0.0, 1.0, 0.0], [0.0, 1.0, 0.0], [0.0, 1.0, 0.0], [0.0, 1.0, 0.0], [0.0, 1.0, 0.0], [0.0, 1.0, 0.0], [0.0, 1.0, 0.0], [0.0, 1.0, 0.0], [0.0, 1.0, 0.0], [0.0, 1.0, 0.0], [0.0, 1.0, 0.0], [0.0, 1.0, 0.0], [0.0, 1.0, 0.0], [0.0, 1.0, 0.0], [0.0, 1.0, 0.0], [0.0, 1.0, 0.0], [0.0, 1.0, 0.0], [0.0, 1.0, 0.0], [0.0, 1.0, 0.0], [0.0, 1.0, 0.0], [0.0, 1.0, 0.0], [0.0, 1.0, 0.0], [0.0, 1.0, 0.0], [0.0, 1.0, 0.0], [0.0, 1.0, 0.0], [0.0, 1.0, 0.0], [0.0, 1.0, 0.0], [0.0, 1.0, 0.0], [0.0, 1.0, 0.0], [0.0, 1.0, 0.0], [0.0, 1.0, 0.0]], "Modul3/AI koeff"=[[0.0, 1.0, 0.0], [0.0, 1.0, 0.0], [0.0, 1.0, 0.0], [0.0, 1.0, 0.0], [0.0, 1.0, 0.0], [0.0, 1.0, 0.0], [0.0, 1.0, 0.0], [0.0, 1.0, 0.0], [0.0, 1.0, 0.0], [0.0, 1.0, 0.0], [0.0, 1.0, 0.0], [0.0, 1.0, 0.0], [0.0, 1.0, 0.0], [0.0, 1.0, 0.0], [0.0, 1.0, 0.0], [0.0, 1.0, 0.0], [0.0, 1.0, 0.0], [0.0, 1.0, 0.0], [0.0, 1.0, 0.0], [0.0, 1.0, 0.0], [0.0, 1.0, 0.0], [0.0, 1.0, 0.0], [0.0, 1.0, 0.0], [0.0, 1.0, 0.0], [0.0, 1.0, 0.0], [0.0, 1.0, 0.0], [0.0, 1.0, 0.0], [0.0, 1.0, 0.0], [0.0, 1.0, 0.0], [0.0, 1.0, 0.0], [0.0, 1.0, 0.0], [0.0, 1.0, 0.0]], "Traps/MachKoeff"=[[0.0, 1.0, 0.0], [-249.333, 111.873, 2.1471], [0.0, 1.0, 0.0], [-249.333, 111.873, 2.1471], [-237.2852, 153.1621, 6.0782], [-237.2852, 153.1621, 6.0782]], "AIsNamen"=["T-MainCol3", "T-Trap1", "T-Trap2", "T-Stirling", "T-PreCol1", "T-PreCol2", "T-MainCol1", "T-MainCol2", "T-T-Line2", "T-MI1", "T-MI2", "T-MI3", "T-MI4", "T-MI5", "T-MI6", "F-MFM1", "T-MainCol4", "T-BHorst1", "T-BHorst2", "T-BHorst3", "T-BHorst4", "T-Oven1", "T-Oven2", "T-T-Line1", "F-MFM2", "P-Me-HP", "P-Me-LP", "P-Vac", "Ref-Turbo", "I-MS-AC", "I-Trap1", "I-Trap2", "Mod2/AI0", "Mod2/AI1", "Mod2/AI2", "Mod2/AI3", "Mod2/AI4", "Mod2/AI5", "Mod2/AI6", "Mod2/AI7", "Mod2/AI8", "Mod2/AI9", "Mod2/AI10", "Mod2/AI11", "Mod2/AI12", "Mod2/AI13", "Mod2/AI14", "Mod2/AI15", "Mod2/AI16", "Mod2/AI17", "Mod2/AI18", "Mod2/AI19", "Mod2/AI20", "Mod2/AI21", "Mod2/AI22", "Mod2/AI23", "Mod2/AI24", "Mod2/AI25", "Mod2/AI26", "Mod2/AI27", "Mod2/AI28", "Mod2/AI29", "Mod2/AI30", "Mod2/AI31", "Mod3/AI0", "Mod3/AI1", "Mod3/AI2", "Mod3/AI3", "Mod3/AI4", "Mod3/AI5", "Mod3/AI6", "Mod3/AI7", "Mod3/AI8", "Mod3/AI9", "Mod3/AI10", "Mod3/AI11", "Mod3/AI12", "Mod3/AI13", "Mod3/AI14", "Mod3/AI15", "Mod3/AI16", "Mod3/AI17", "Mod3/AI18", "Mod3/AI19", "Mod3/AI20", "Mod3/AI21", "Mod3/AI22", "Mod3/AI23", "Mod3/AI24", "Mod3/AI25", "Mod3/AI26", "Mod3/AI27", "Mod3/AI28", "Mod3/AI29", "Mod3/AI30", "Mod3/AI31"], "DIOsMod0Name"=["blindDIO0"], "DIOsMod1Name"=["on/off P-MS", "MS Start", "MS Stop", "FanMach1", "FanReserve", "Valve1A", "on/off PrePump", "S1Reserve", "on/off VacP2", "on/off VacP1", "S1D", "FanMach2", "S1C", "on/off Stirling", "S1B", "S1A", "Valve1B", "on/off Turbo"], "DIOsMod2AName"=["blindDIO2A"], "DIOsMod2BName"=["blindDIO2B"], "HorstMod0Name"=["MFC1B"], "HorstMod1Name"=["PressContr1A", "PressContr1B", "PressContr1C"], "HorstMod2AName"=["MFC1A"], "HorstMod2BName"=["PressContr1D"], "Startmethode"=0, "Dateiordner Housekeeping"=path "C:/", "Dateiname Housekeeping"="test"} ("Einstellungen")
  n1 = Open/Create/Replace File(file path (use dialog)=path "c:/einstellungen.per" ("Datei (Dialog verwenden)"), operation (0:open)=T3."open" ("Operation (0:Öffnen)")) -> (refnum out=w11:refnum<file>)  [unwired: 4 in, 2 out]
  n2 = Read from Binary File(5:T2 {"DIOsMod0Nr"=[], "DIOsMod1Nr"=[], "DIOsMod2ANr"=[], "DIOsMod2BNr"=[], "AIsLH"=[], "Anzahl Horst/Modul"=[], "Regler für den Probenfluß"=0, "StringSPvorgebenMod0"=[], "StringSPvorgebenMod1"=[], "StringSPvorgebenMod2A"=[], "StringSPvorgebenMod2B"=[], "StringMWAntwort0"=[], "StringMWAntwort1"=[], "StringMWAntwort2A"=[], "StringMWAntwort2B"=[], "UmrechnungHorst0"=[], "UmrechnungHorst1"=[], "UmrechnungHorst2A"=[], "UmrechnungHorst2B"=[], "StringMWabfragenMod0"=[], "StringMWabfragenMod1"=[], "StringMWabfragenMod2A"=[], "StringMWabfragenMod2B"=[], "Modul1/AI koeff"=[], "Modul2/AI koeff"=[], "Modul3/AI koeff"=[], "Traps/MachsKoeff"=[], "Modul1/AIsNamen"=[], "Modul2/AIsNamen"=[], "Modul3/AIsNamen"=[], "DIOsMod0Name"=[], "DIOsMod1Name"=[], "DIOsMod2AName"=[], "DIOsMod2BName"=[], "HorstMod0Name"=[], "HorstMod1Name"=[], "HorstMod2AName"=[], "HorstMod2BName"=[], "Startmethode"=0, "Dateiordner Housekeeping"=path "", "Dateiname Housekeeping"="", "DateiordnerECD1"=path "", "DateinameECD1"="", "DateiordnerECD2"=path "", "DateinameECD2"="", "NamenLangsameHeizungen"=[], "ModuleLH"=[]} ("Einstellungen"), 11:w11) -> (2:w9:T2, 3:w10:refnum<file>)  [unwired: 4 in, 2 out]
  n3 = Close File(refnum=w10) -> ()  [unwired: 1 in, 2 out]
  n4 = flat-sequence {
    tunnel: [w125] -> w45
    tunnel: [w46] -> w44
    tunnel: [w152] -> w40
    tunnel: [w149] -> w39
    tunnel: [w151] -> w38
    tunnel: [w141] -> w37
    tunnel: [w150] -> w36
    tunnel: [w50] -> w35
    tunnel: [w140] -> w34
    tunnel: [w139] -> w33
    tunnel: [w132] -> w32
    tunnel: [w54] -> w31
    tunnel: [w95] -> w30
    tunnel: [w148] -> w29
    tunnel: [w138] -> w28
    tunnel: [w137] -> w27
    tunnel: [w128] -> w26
    tunnel: [w127] -> w25
    tunnel: [w126] -> w24
    tunnel: [w124] -> w23
    tunnel: [w123] -> w22
    tunnel: [w122] -> w21
    tunnel: [w119] -> w20
    tunnel: [w101] -> w15
    tunnel: w9 -> [w49]
    tunnel: [w94] -> w14
    tunnel: w3 -> [w100]
    tunnel: [w46] -> w1
    tunnel: w45 -> [w171]
    tunnel: w44 -> [w256]
    tunnel: [w255] -> w43
    tunnel: [w254] -> w42
    tunnel: [w171] -> w41
    tunnel: w40 -> [_]
    tunnel: w39 -> [w207]
    tunnel: w38 -> [w206]
    tunnel: w37 -> [w208]
    tunnel: w36 -> [w205]
    tunnel: w35 -> [w175]
    tunnel: w34 -> [w170]
    tunnel: w33 -> [w165]
    tunnel: w32 -> [w162]
    tunnel: w31 -> [w163]
    tunnel: w30 -> [w166]
    tunnel: w29 -> [w252]
    tunnel: w28 -> [w173]
    tunnel: w27 -> [w253]
    tunnel: w26 -> [w250]
    tunnel: w25 -> [w249]
    tunnel: w24 -> [w248]
    tunnel: w23 -> [w247]
    tunnel: w22 -> [w246]
    tunnel: w21 -> [w245]
    tunnel: w20 -> [w197]
    tunnel: [w184] -> w19
    tunnel: [w183] -> w18
    tunnel: [w182] -> w17
    tunnel: [w181] -> w16
    tunnel: w15 -> [w174]
    tunnel: w14 -> [w161]
    tunnel: w3 -> [w160]
    tunnel: w1 -> [w158]
    tunnel: w43 -> [w867]
    tunnel: w42 -> [w866]
    tunnel: w41 -> [w865]
    tunnel: w19 -> [w862]
    tunnel: w18 -> [w861]
    tunnel: w17 -> [w860]
    tunnel: w16 -> [w859]
    frame #0 {
      w144 = string[] ["U_WiderstandTrap1 [V]", "TemperaturTrap1 [°C]", "U_WiderstandTrap2 [V]", "TemperaturTrap2 [°C]", "TemperaturMach1 [°C]", "TemperaturMach2 [°C]"]
      w146 = string[] ["Big Ben [s]", "Methodenzeit [s]", "Zykluszeit [s] Mod0", "Zykluszeit [s] Mod1", "Zykluszeit [s] Mod2A", "Zykluszeit [s] Mod2B"]
      w133 = FALSE ("Undefinierte Werte möglich")
      w135 = FALSE ("global stop RT")
      n5 = Unbundle(w49) -> ("DIOsMod0Nr"=w99:i32[], "DIOsMod1Nr"=w98:i32[], "DIOsMod2ANr"=w97:i32[], "DIOsMod2BNr"=w96:i32[], "AIsLH"=w51:i32[], "Anzahl Horst/Modul"=w95:i32[], "Regler für den Probenfluß"=w94:i32, "StringSPvorgebenMod0"=w93:string[], "StringSPvorgebenMod1"=w92:string[], "StringSPvorgebenMod2A"=w91:string[], "StringSPvorgebenMod2B"=w90:string[], "StringMWAntwort0"=w89:string[], "StringMWAntwort1"=w88:string[], "StringMWAntwort2A"=w87:string[], "StringMWAntwort2B"=w86:string[], "UmrechnungHorst0"=w85:dbl[], "UmrechnungHorst1"=w84:dbl[], "UmrechnungHorst2A"=w83:dbl[], "UmrechnungHorst2B"=w82:dbl[], "StringMWabfragenMod0"=w81:string[], "StringMWabfragenMod1"=w80:string[], "StringMWabfragenMod2A"=w79:string[], "StringMWabfragenMod2B"=w78:string[], "Modul1/AI koeff"=w77:dbl[][], "Modul2/AI koeff"=w76:dbl[][], "Modul3/AI koeff"=w75:dbl[][], "Traps/MachsKoeff"=w74:dbl[][], "Modul1/AIsNamen"=w73:string[], "Modul2/AIsNamen"=w72:string[], "Modul3/AIsNamen"=w71:string[], "DIOsMod0Name"=w69:string[], "DIOsMod1Name"=w68:string[], "DIOsMod2AName"=w67:string[], "DIOsMod2BName"=w66:string[], "HorstMod0Name"=w65:string[], "HorstMod1Name"=w64:string[], "HorstMod2AName"=w63:string[], "HorstMod2BName"=w62:string[], "Startmethode"=w46:i32, "Dateiordner Housekeeping"=w61:path, "Dateiname Housekeeping"=w60:string, "DateiordnerECD1"=w59:path, "DateinameECD1"=w58:string, "DateiordnerECD2"=w57:path, "DateinameECD2"=w56:string, "NamenLangsameHeizungen"=w55:string[], "ModuleLH"=w48:i32[])
      n6 = global write "gvbooleschRT.vi" "global stop RT"(w135) -> ()
      n7 = Decrement(x=w48) -> (x-1=w47:i32[])
      n8 = Multiply(x=w47, y=32) -> (x*y=w52:i32[])
      n9 = property on="dargestellte Größe 2" class="Ring (strict)"("AllowUndefVals"=w133) -> ()  [unwired: 2 in, 2 out]
      n10 = property on="Zeitachse2" class="Ring (strict)"("AllowUndefVals"=w133) -> ()  [unwired: 2 in, 2 out]
      n11 = property on="Zeitachse1" class="Ring (strict)"("AllowUndefVals"=w133) -> ()  [unwired: 2 in, 2 out]
      n12 = property on="dargestellte Größe 1" class="Ring (strict)"("AllowUndefVals"=w133) -> ()  [unwired: 2 in, 2 out]
      n13 = property on="Methode" class="Ring (strict)"("AllowUndefVals"=w133) -> ()  [unwired: 2 in, 2 out]
      n14 = property on="Methode" class="Ring (strict)"("Value"=w46) -> ()  [unwired: 2 in, 2 out]
      n15 = Add(x=w52, y=w51) -> (x+y=w50:i32[])
      n16 = for {
        tunnel: [w153] -> w142 mode=indexing
        tunnel: w100 -> [w154] mode=indexing
        n17 = Unbundle(w154) -> ("Methodenname"=w153:string)  [unwired: 40 out]
      }
      n18 = local write "global stop RT"(w135) -> ()
      n19 = call "FPGA-Start.vi"() -> ("error out"=w152:errorcluster, "FPGA VI Reference Out"=w125:refnum<k20>)  [unwired: 2 in]
      n20 = Build Array (concatenate)(w73, w72, w71) -> (w70:string[])
      n21 = property on="Methode" class="Ring (strict)"("Strings []"=w142) -> ()  [unwired: 2 in, 2 out]
      n22 = Open/Create/Replace File(file path (use dialog)=path "c:/fromcriocmd.txt" ("Pfad MS-Datei CRIO"), operation (0:open)=T3."replace or create" ("Operation (0:Öffnen)")) -> (refnum out=w110:refnum<file>, error out=w109:errorcluster)  [unwired: 4 in, 1 out]
      n23 = Open/Create/Replace File(file path (use dialog)=path "c:/fromcriordy.txt" ("Dateipfad (Dialog verwenden)"), operation (0:open)=T3."replace or create" ("Operation (0:Öffnen)")) -> (refnum out=w104:refnum<file>, error out=w105:errorcluster)  [unwired: 4 in, 1 out]
      n24 = Write to Text File(file (use dialog)=w110, text="time=              \ncycle=   \ninfo=                                                                                                                                                      \nlength=   \ncmd=" ("Text0 MS-Datei"), error in=w109) -> (refnum out=w107:refnum<file>, error out=w106:errorcluster)  [unwired: 1 in, 1 out]
      n25 = Close File(refnum=w104, error in=w105) -> (path=w138:path)  [unwired: 1 out]
      n26 = Close File(refnum=w107, error in=w106) -> (path=w101:path)  [unwired: 1 out]
      n27 = call "TDMS0.vi"("Startmethode"=w46, "Dateiname"=w58, "Dateiordner"=w59) -> ("tdms1"=w115:refnum<k34>, "tdms0"=w116:refnum<k34>)
      n28 = call "TDMS0.vi"("Startmethode"=w46, "Dateiname"=w60, "Dateiordner"=w61) -> ("tdms1"=w117:refnum<k34>, "tdms0"=w118:refnum<k34>)
      n29 = call "TDMS0.vi"("Startmethode"=w46, "Dateiname"=w56, "Dateiordner"=w57) -> ("tdms1"=w113:refnum<k34>, "tdms0"=w114:refnum<k34>)
      n30 = Build Array (concatenate)(w65, w64, w63, w62) -> (w143:string[])
      n31 = Build Array (concatenate)(w93, w92, w91, w90) -> (w151:string[])
      n32 = Build Array (concatenate)(w81, w80, w79, w78) -> (w149:string[])
      n33 = global write "GVaktuelleTDMS.vi" "aktuelleTDMS-DateiECD2"(w114) -> ()
      n34 = global write "GVaktuelleTDMS.vi" "aktuelleTDMS-DateiECD1"(w116) -> ()
      n35 = global write "GVaktuelleTDMS.vi" "aktuelleTDMS-DateiHK"(w118) -> ()
      n36 = Build Array (concatenate)(w89, w88, w87, w86) -> (w150:string[])
      n37 = Add Array Elements(numeric array=w95) -> (sum=w132:i32)
      n38 = Build Array (concatenate)(w85, w84, w83, w82) -> (w141:dbl[])
      n39 = Split 1D Array(array=w146, index=2 ("Index")) -> (second subarray=w136:string[])  [unwired: 1 out]
      n40 = property on="Zeitachse1" class="Ring (strict)"("Strings []"=w136) -> ()  [unwired: 2 in, 2 out]
      n41 = property on="Zeitachse2" class="Ring (strict)"("Strings []"=w136) -> ()  [unwired: 2 in, 2 out]
      n42 = Build Array (concatenate)(w70, w144, w143) -> (w134:string[])
      n43 = Index Array(array=w74, index (col)=2 ("Deaktivierter Index (Spalte)")) -> (element=w128:dbl[])  [unwired: 1 in]
      n44 = Index Array(array=w74, index (col)=1 ("Deaktivierter Index (Spalte)")) -> (element=w127:dbl[])  [unwired: 1 in]
      n45 = Index Array(array=w74, index (col)=0 ("Deaktivierter Index (Spalte)")) -> (element=w126:dbl[])  [unwired: 1 in]
      n46 = call "AIKoeffSortieren.vi"("Modul3/AI koeff"=w75, "Modul2/AI koeff"=w76, "Modul1/AI koeff"=w77) -> ("P0"=w122:dbl[], "P1"=w123:dbl[], "P2"=w124:dbl[])
      n47 = Build Cluster Array(w99, w98, w97, w96) -> (w140:cluster{"DIOsMod2BNr":i32[]}[])
      n48 = for {
        tunnel: w140 -> [w156] mode=indexing
        tunnel: [w157] -> w139 mode=indexing
        n49 = Unbundle(w156) -> ("DIOsMod2BNr"=w155:i32[])
        n50 = Array Size(array=w155) -> (size(s)=w157:i32)
      }
      n51 = property on="dargestellte Größe 1" class="Ring (strict)"("Strings []"=w134) -> ()  [unwired: 2 in, 2 out]
      n52 = property on="dargestellte Größe 2" class="Ring (strict)"("Strings []"=w134) -> ()  [unwired: 2 in, 2 out]
      n53 = Bundle("DIOsMod0Name"=w69, "DIOsMod1Name"=w68, "DIOsMod2AName"=w67, "DIOsMod2BName"=w66, "HorstMod0Name"=w65, "HorstMod1Name"=w64, "HorstMod2AName"=w63, "HorstMod2BName"=w62, "NamenLangsameHeizungen"=w55) -> (w137:T10)  [unwired: 1 in]
      n54 = Build Array (concatenate)(string[] ["Datei Nr.", "Zyklusnr. Mod0", "Zyklusnr. Mod1", "Zyklusnr. Mod2A", "Zyklusnr. Mod2B"], w146, w70, w144, w143, "Probenvolumen1", "Probenvolumen2") -> (w148:string[])
      n55 = Bundle("Dateiordner Housekeeping"=w61, "DateiordnerECD1"=w59, "DateiordnerECD2"=w57, "Dateiname Housekeeping"=w60, "DateinameECD1"=w58, "DateinameECD2"=w56, "tdms0"=w118, "tdms1"=w117, "tdms0"=w116, "tdms1"=w115, "tdms0"=w114, "tdms1"=w113) -> (w119:T11)  [unwired: 1 in]
      n56 = Array Size(array=w55) -> (size(s)=w54:i32)
    }
    frame #1 {
      w224 = 0
      w222 = string[] []
      w198 = 0 ("Zyklusnummer1")
      n57 = while {
        shift-right: ["Methode"] -> _
        shift-left: w256 -> [w856]
        stop <- w858 stop-if-true
        n58 = call "Bis zum nächsten Vielfachen warten7"("Count(mSec)"=u32 1000) -> ()  [unwired: 1 out]
        n59 = Not Equal?(x=w856, y="Methode") -> (x != y?=w854:bool)
        n60 = global write "GVMethodenwechsel.vi" "Methodenwechsel?"(w854) -> ()
        n61 = global read "gvbooleschRT.vi" "global stop RT"() -> (w858:bool)
      }
      n62 = Add Array Elements(numeric array=w165) -> (sum=w164:i32)
      n63 = Array Size(array=w175) -> (size(s)=w201:i32)
      n64 = Index Array(array=w160, index=w158) -> (element=w159:T12)
      n65 = while {
        stop <- w827 stop-if-true
        w821 = 10.0
        n66 = global read "GVTrapsMachs.vi" "Traps/Machs"() -> (w817:dbl[])
        n67 = global read "GVAIs.vi" "AIs"() -> (w818:dbl[])
        n68 = call "Bis zum nächsten Vielfachen warten"("Count(mSec)"=u32 1000) -> ()  [unwired: 1 out]
        n69 = for {
          N: 9 -> [_]
          shift-right: [w830] -> w824
          shift-left: w818 -> [w831]
          shift-right: [w828] -> w822
          shift-left: w817 -> [w829]
          n70 = flat-sequence {
            tunnel: w831 -> [w838]
            tunnel: [w837] -> w830
            tunnel: w829 -> [w836]
            tunnel: [w835] -> w828
            frame #0 {
              n71 = call "Warten28"("Count(mSec)"=u32 100) -> ()  [unwired: 1 out]
            }
            frame #1 {
              n72 = global read "GVTrapsMachs.vi" "Traps/Machs"() -> (w833:dbl[])
              n73 = global read "GVAIs.vi" "AIs"() -> (w834:dbl[])
              n74 = Add(x=w838, y=w834) -> (x+y=w837:dbl[])
              n75 = Add(x=w833, y=w836) -> (x+y=w835:dbl[])
            }
          }
        }
        n76 = Divide(x=w824, y=w821) -> (x/y=w823:dbl[])
        n77 = Divide(x=w822, y=w821) -> (x/y=w820:dbl[])
        n78 = Build Array (concatenate)(w823, w820) -> (w819:dbl[])
        n79 = global write "GVHK1Hz.vi" "Mod1Mod2Mod3/AITrapsMachs1Hz"(w819) -> ()
        n80 = global read "gvbooleschRT.vi" "global stop RT"() -> (w827:bool)
      }
      n81 = while {
        tunnel: w171 -> [w329]
        tunnel: w247 -> [w328]
        tunnel: w246 -> [w327]
        tunnel: w245 -> [w326]
        stop <- w330 stop-if-true
        n82 = call "AIsFIFORT.vi"("P0"=w326, "P1"=w327, "P2"=w328, "FPGA VI Reference In"=w329) -> (0:w325)
        n83 = global read "gvbooleschRT.vi" "global stop RT"() -> (w330:bool)
        n84 = global write "GVAIs.vi" "AIs"(w325) -> ()
      }
      n85 = Initialize Array(cluster{"output high":dbl, "output low":dbl} {"output high"=99999.0, "output low"=0.0} ("output range"), w201) -> (w176:cluster{"output high":dbl, "output low":dbl}[])
      n86 = while {
        tunnel: w171 -> [w332]
        tunnel: w250 -> [w336]
        tunnel: w249 -> [w334]
        tunnel: w248 -> [w333]
        stop <- w337 stop-if-true
        n87 = call "TrapsMachMitteln.vi"("Traps/MachKoeff0"=w333, "Traps/MachKoeff1"=w334, "Traps/MachKoeff2"=w336, "FPGA VI Reference In"=w332) -> (0:w331)
        n88 = global read "gvbooleschRT.vi" "global stop RT"() -> (w337:bool)
        n89 = call "Bis zum nächsten Vielfachen warten16"("Count(mSec)"=u32 100) -> ()  [unwired: 1 out]
        n90 = global write "GVTrapsMachs.vi" "Traps/Machs"(w331) -> ()
      }
      n91 = Initialize Array(-1 ("Element"), 4 ("Dimension")) -> (w167:i32[])
      n92 = while {
        tunnel: w253 -> [w460]
        shift-right: [w459] -> _
        shift-left: w160 -> [w437]
        tunnel: w176 -> [w458]
        tunnel: w175 -> [w457]
        tunnel: w171 -> [w456]
        tunnel: w174 -> [w455]
        tunnel: w173 -> [w454]
        shift-right: [w446] -> _
        shift-left: 0 -> [w453]
        tunnel: w171 -> [w452]
        tunnel: w170 -> [w451]
        shift-right: [w445] -> _
        shift-left: 0.0 -> [w450]
        shift-right: [w444] -> _
        shift-left: -1 -> [w449]
        shift-right: [w443] -> _
        shift-left: w167 -> [w448]
        tunnel: w166 -> [w438]
        tunnel: w165 -> [w439]
        tunnel: w164 -> [w440]
        tunnel: w163 -> [w441]
        tunnel: w162 -> [w442]
        tunnel: w161 -> [w447]
        shift-right: [w358] -> _
        shift-left: w159 -> [w357]
        i -> [w361]
        stop <- w461 stop-if-true
        w403 = FALSE
        w402 = 0.0
        w404 = 0  # ZeilennummerMPV
        w408 = cluster{dbl[], dbl[]} {[], []}
        w418 = dbl[] []
        w422 = 0  # ZeileMach2
        w423 = 0  # ZeileMach1
        w424 = 0  # ZeileFPGAFixp
        w425 = 0  # ZeileFPGAPID
        w426 = 0  # ZeileFPGABoolesch
        w427 = i32[] [0, 0, 0, 0]  # ZeilennummernHorst
        w428 = i32[] [0, 0, 0, 0]  # ZeilennummernDIOs
        n93 = local read "Methode"() -> (w360:i32)
        n94 = Index Array(array=w437, index=w360) -> (element=w359:T12)
        n95 = Unbundle(w357) -> ("Zykluslängen [s]"=w401:dbl[], "ZeitpktDIOsMod0"=w400:dbl[], "ZeitpktDIOsMod1"=w399:dbl[], "ZeitpktDIOsMod2A"=w398:dbl[], "ZeitpktDIOsMod2B"=w397:dbl[], "DIOsSPMod0"=w396:bool[][], "DIOsSPMod1"=w395:bool[][], "DIOsSPMod2A"=w394:bool[][], "DIOsSPMod2B"=w393:bool[][], "Mod0HorstZeitpkt"=w392:dbl[], "Mod1HorstZeitpkt"=w391:dbl[], "Mod2AHorstZeitpkt"=w390:dbl[], "Mod2BHorstZeitpkt"=w389:dbl[], "HorstSPMod0"=w388:dbl[][], "HorstSPMod1"=w387:dbl[][], "HorstSPMod2A"=w386:dbl[][], "HorstSPMod2B"=w385:dbl[][], "LangsameHeizungenSP"=w384:dbl[], "LHHeizen?"=w383:bool[], "ZPktFPGABoolesch"=w382:dbl[], "FPGABoolesch"=w381:bool[][], "ZeitpktFPGAPID"=w380:dbl[], "FPGAPID"=w379:T13, "ZeitpktFPGAFixp"=w378:dbl[], "FPGAFixp"=w377:fxp<+/-,16,4>[][], "ZeitpktMach1"=w376:dbl[], "TempMach1"=w375:dbl[], "ZeitpktMach2"=w374:dbl[], "TempMach2"=w373:dbl[], "PIDs für \"träge\" Heizungen"=w372:T14, "Zwangsbedingungen"=w371:dbl[][], "Dateien fürs MS schicken?"=w370:bool, "ZeitpunkteMPV"=w369:dbl[], "SPMPV"=w368:i32[], "ZeitpktMSa"=w367:dbl, "ZeitpktMSb"=w366:dbl, "Int.Start1"=w365:dbl, "Int.Stop1"=w364:dbl, "Int.Start2"=w363:dbl, "Int.Stop2"=w362:dbl)  [unwired: 1 out]
        "Zykluslängen [s]" <- w401
        n96 = Add(x=w448, y=1) -> (x+y=w412:i32[])
        n97 = Add(x=w449, y=1) -> (x+y=w434:i32)
        n98 = global read "GVaktuelleTDMS.vi" "aktuelleTDMS-DateiECD1"() -> (w410:refnum<k34>)
        n99 = global read "GVZwangs.vi" "ZwangsFPGABoolesch?"() -> (w415:bool[])
        n100 = global read "GVZeitenZyklen.vi" "ZyklusNummern"() -> (w411:i32[])
        n101 = global read "GVZwangs.vi" "ZwangsHorst?"() -> (w417:cluster{bool[]}[])
        n102 = global read "GVZwangs.vi" "ZwangsDIO?"() -> (w416:cluster{bool[]}[])
        n103 = while {
          tunnel: w439 -> [w613]
          tunnel: w442 -> [w611]
          tunnel: w441 -> [w610]
          tunnel: w438 -> [w612]
          tunnel: w440 -> [w609]
          tunnel: w371 -> [w601]
          stop <- w603 stop-if-true
          n104 = local read "Methode"() -> (w608:i32)
          n105 = global read "gvbooleschRT.vi" "global stop RT"() -> (w606:bool)
          n106 = case shown="True" "global stop RT" {
            frame False {
            }
            frame True {
              n107 = global write "gvbooleschRT.vi" "global stop RT"(TRUE ("global stop RT")) -> ()
            }
          }
          n108 = call "ZwangsbedingungenGV.vi"("AnzahlHorst"=w611, "AnzahlHorst/Modul"=w612, "AnzahlLH"=w610, "AnzahlDIOs/Modul"=w613, "AnzahlDIOs"=w609, "Zwangsbedingungen"=w601, "Methodennummer"=w608) -> ("Methodennummer"=w607:i32)  [unwired: 4 in]
          n109 = local read "veränderte Methode benutzen"() -> (w604:bool)
          n110 = global read "GVMethodenwechsel.vi" "Methodenwechsel?"() -> (w605:bool)
          n111 = local write "Methode"(w607) -> ()
          n112 = Compound Arithmetic op=OR(w606, w605, w604) -> (w603:bool)
          n113 = call "Bis zum nächsten Vielfachen warten10"("Count(mSec)"=u32 1000) -> ()  [unwired: 1 out]
        }
        n114 = while {
          tunnel: w457 -> [w524]
          tunnel: w458 -> [w525]
          tunnel: w456 -> [w521]
          tunnel: w384 -> [w515]
          tunnel: w372 -> [w514]
          stop <- w510 stop-if-true
          n115 = global read "GVAIs.vi" "AIs"() -> (w516:dbl[])
          n116 = call "Bis zum nächsten Vielfachen warten12"("Count(mSec)"=u32 100) -> ()  [unwired: 1 out]
          n117 = for {
            tunnel: w516 -> [w600]
            tunnel: w524 -> [w599] mode=indexing
            tunnel: [w598] -> w523 mode=indexing
            n118 = Index Array(array=w600, index=w599) -> (element=w598:dbl)
          }
          n119 = global read "gvbooleschRT.vi" "global stop RT"() -> (w513:bool)
          n120 = local read "veränderte Methode benutzen"() -> (w511:bool)
          n121 = global read "GVMethodenwechsel.vi" "Methodenwechsel?"() -> (w512:bool)
          n122 = call-poly <vilib>:"PID.vi"("output range"=w525, "PID gains"=w514, "process variable"=w523, "setpoint"=w515) -> ("output"=w522:dbl[])  [unwired: 6 in, 1 out]
          n123 = global read "GVHeizenLH.vi" "Heizen?LH"() -> (w517:bool[])
          n124 = Compound Arithmetic op=OR(w513, w512, w511) -> (w510:bool)
          n125 = To Unsigned Long Integer(number=w522) -> (unsigned 32bit integer=w519:u32[])
          n126 = Array To Cluster(array=w517) -> (cluster=w520:T15)
          n127 = Array To Cluster(array=w519) -> (cluster=w518:T16)
          n128 = xnode "Read/Write Control"("FPGA VI Reference In"=w521, "LHHeizen?"=w520, "LHPulse(us)"=w518) -> ()  [unwired: 1 in, 2 out]
        }
        n129 = while {
          tunnel: w460 -> [w793]
          shift-right: [w784] -> _
          shift-left: w359 -> [w792]
          tunnel: w360 -> [w790]
          shift-right: [w782] -> w459
          shift-left: w437 -> [w791]
          tunnel: [w783] -> w358
          stop <- w786 stop-if-true
          n130 = global read "GVMethodenwechsel.vi" "Methodenwechsel?"() -> (w788:bool)
          n131 = global read "gvbooleschRT.vi" "global stop RT"() -> (w787:bool)
          n132 = case shown="True" "Methode verändern" {
            tunnel: w793 -> [_ w815]
            tunnel: w792 -> [w812 w814]
            tunnel: [w812 w813] -> w784
            frame False {
            }
            frame True {
              n133 = call "methodeändern.vi"("Methode"=w814, "Namen"=w815) -> ("Methode"=w813:T12)  [unwired: 1 in]
              n134 = property on="Methode verändern" class="Bool (strict)"("Value"=FALSE ("Methode verändern")) -> ()  [unwired: 2 in, 2 out]
            }
          }
          n135 = Compound Arithmetic op=OR(w788, w787, "veränderte Methode benutzen") -> (w786:bool)
          n136 = case shown="True" "Methode speichern" {
            tunnel: w784 -> [_ w809]
            tunnel: w791 -> [w802 w811]
            tunnel: w790 -> [_ w810]
            tunnel: [w802 w804] -> w782
            frame False {
            }
            frame True {
              n137 = Replace Array Subset(array=w811, new element=w809, index=w810) -> (w804:T1)
              n138 = property on="Methode speichern" class="Bool (strict)"("Value"=FALSE ("Methode speichern")) -> ()  [unwired: 2 in, 2 out]
              n139 = Open/Create/Replace File(file path (use dialog)=path "c:/methoden.per" ("Dateipfad (Dialog verwenden)"), operation (0:open)=T3."replace" ("Operation (0:Öffnen)")) -> (refnum out=w806:refnum<file>)  [unwired: 4 in, 2 out]
              n140 = Write to Binary File(file (use dialog)=w806, data=w804) -> (refnum out=w803:refnum<file>)  [unwired: 4 in, 2 out]
              n141 = Close File(refnum=w803) -> ()  [unwired: 1 in, 2 out]
            }
          }
          n142 = case shown="False" "veränderte Methode benutzen" {
            tunnel: w784 -> [_ w799]
            tunnel: [w796 w799] -> w783
            tunnel: w782 -> [w798 _]
            frame False {
              n143 = local read "Methode"() -> (w797:i32)
              n144 = Index Array(array=w798, index=w797) -> (element=w796:T12)
            }
            frame True {
              n145 = flat-sequence {
                frame #0 {
                  n146 = call "Warten"("Count(mSec)"=u32 1100) -> ()  [unwired: 1 out]
                }
                frame #1 {
                  n147 = property on="veränderte Methode benutzen" class="Bool (strict)"("Value"=FALSE ("Methode verändern")) -> ()  [unwired: 2 in, 2 out]
                }
              }
            }
          }
          n148 = call "Bis zum nächsten Vielfachen warten8"("Count(mSec)"=u32 500) -> ()  [unwired: 1 out]
        }
        n149 = Build Cluster Array(w396, w395, w394, w393) -> (w432:cluster{"DIOsSPMod2B":bool[][]}[])
        n150 = Build Cluster Array(w388, w387, w386, w385) -> (w430:cluster{"HorstSPMod2B":dbl[][]}[])
        n151 = Bundle(w418, w418, w418, w418) -> (w419:cluster{dbl[], dbl[], dbl[], dbl[]})  [unwired: 1 in]
        n152 = Build Cluster Array(w400, w399, w398, w397) -> (w433:cluster{"ZeitpktDIOsMod2B":dbl[]}[])
        n153 = Build Cluster Array(w392, w391, w390, w389) -> (w431:cluster{"Mod2BHorstZeitpkt":dbl[]}[])
        n154 = Equal?(x=w361, y=0) -> (x = y?=w435:bool)
        n155 = while {
          shift-right: [w474] -> _
          shift-left: w403 -> [w478]
          shift-right: [w473] -> _
          shift-left: w402 -> [w477]
          shift-right: [w472] -> _
          shift-left: w403 -> [w476]
          shift-right: [w471] -> _
          shift-left: w402 -> [w475]
          tunnel: w447 -> [w470]
          tunnel: w365 -> [w465]
          tunnel: w364 -> [w464]
          tunnel: w363 -> [w463]
          tunnel: w362 -> [w462]
          stop <- w467 stop-if-true
          n156 = call "Integrieren.vi"("Integrieren1"=w478, "Integral1"=w477, "Integrieren2"=w476, "Integral2"=w475, "Int.Start1"=w465, "Int.Stop1"=w464, "Int.Start2"=w463, "HorstProbenflußNr."=w470, "Int.Stop2"=w462) -> ("Integrieren1"=w474:bool, "Integral1"=w473:dbl, "Integrieren2"=w472:bool, "Integral2"=w471:dbl)  [unwired: 7 in]
          n157 = global read "gvbooleschRT.vi" "global stop RT"() -> (w469:bool)
          n158 = local read "veränderte Methode benutzen"() -> (w466:bool)
          n159 = global read "GVMethodenwechsel.vi" "Methodenwechsel?"() -> (w468:bool)
          n160 = Compound Arithmetic op=OR(w469, w468, w466) -> (w467:bool)
          n161 = call "Bis zum nächsten Vielfachen warten9"("Count(mSec)"=u32 100) -> ()  [unwired: 1 out]
        }
        n162 = Bundle(w433, w432, w431, w430, "LHHeizen?"=w383, "ZPktFPGABoolesch"=w382, "FPGABoolesch"=w381, "ZeitpktFPGAPID"=w380, "FPGAPID"=w379, "ZeitpktFPGAFixp"=w378, "FPGAFixp"=w377, "ZeitpktMach1"=w376, "TempMach1"=w375, "ZeitpktMach2"=w374, "TempMach2"=w373, "ZeitpunkteMPV"=w369, "SPMPV"=w368) -> (w429:T17)  [unwired: 1 in]
        n163 = Bundle("ZyklusNummern"=w411, "ZeilennummernDIOs"=w428, "ZwangsDIO?"=w416, "ZeilennummernHorst"=w427, "ZwangsHorst?"=w417, "ZeileFPGABoolesch"=w426, "ZwangsFPGABoolesch?"=w415, "ZeileFPGAPID"=w425, "ZeileFPGAFixp"=w424, "ZeileMach1"=w423, "ZeileMach2"=w422, "ZeilennummerMPV"=w404) -> (w421:T18)  [unwired: 1 in]
        n164 = while "ZyklusSteuerung" {
          tunnel: w451 -> [w710]
          tunnel: w452 -> [w708]
          shift-right: [w706] -> _
          shift-left: w421 -> [w707]
          tunnel: w429 -> [w709]
          stop <- w702 stop-if-true
          n165 = call "ZyklussteuerungGV.vi"("Zeitpunkte/SPs"=w709, "DIOsNummern"=w710, "Schieberegister"=w707, "FPGA VI Reference In"=w708) -> ("Schieberegister"=w706:T19)  [unwired: 2 in]
          n166 = global read "gvbooleschRT.vi" "global stop RT"() -> (w704:bool)
          n167 = local read "veränderte Methode benutzen"() -> (w703:bool)
          n168 = global read "GVMethodenwechsel.vi" "Methodenwechsel?"() -> (w705:bool)
          n169 = Compound Arithmetic op=OR(w705, w704, w703) -> (w702:bool)
          n170 = call "Bis zum nächsten Vielfachen warten11"("Count(mSec)"=u32 100) -> ()  [unwired: 1 out]
        }
        n171 = while {
          shift-right: [w660] -> _
          shift-left: w419 -> [w667]
          shift-right: [w659] -> _
          shift-left: w419 -> [w666]
          shift-right: [w657] -> _
          shift-left: T7 {"Zyklus1"=0, "Zeitachse1"=0, "dargestellte Größe 1"=0, "Zyklus2"=0, "Zeitachse2"=0, "dargestellte Größe 2"=0} ("AnzeigeEinstellungen") -> [w665]
          tunnel: w401 -> [w632]
          shift-right: [w628] -> _
          shift-left: w410 -> [w627]
          shift-right: [w622] -> _
          shift-left: w408 -> [w624]
          shift-right: [w616] -> _
          shift-left: w408 -> [w623]
          shift-right: ["Detektor"] -> _
          shift-left: 0 ("Detektor") -> [w620]
          stop <- w671 stop-if-true
          w633 = 0.0 ("X-Achse.Bereich:Minimum")
          n172 = case shown="0, Default" "Detektor" {
            tunnel: [w678 w689] -> w622
            tunnel: w632 -> [w677 w692]
            tunnel: "Detektor" -> [w676 w691]
            tunnel: [w675 w690] -> w630
            tunnel: [w674 w688] -> w628
            frame 0, Default {
              n173 = Index Array(array=w677, index=w676) -> (element=w675:dbl)
              n174 = global read "GVaktuelleTDMS.vi" "aktuelleTDMS-DateiECD1"() -> (w674:refnum<k34>)
              n175 = TDMS Read(0:w674, 7:"ECD1", 12:dbl[] []) -> (10:w679:dbl[])  [unwired: 4 in, 5 out]
              n176 = Array Size(array=w679) -> (size(s)=w681:i32)
              n177 = for {
                N: w681 -> [_]
                tunnel: [w684] -> w680 mode=indexing
                i -> [w687]
                n178 = To Double Precision Float(number=w687) -> (double precision float=w686:dbl)
                n179 = Divide(x=w686, y=10.0) -> (x/y=w684:dbl)
              }
              n180 = Bundle(w680, w679) -> (w678:cluster{dbl[], dbl[]})  [unwired: 1 in]
            }
            frame 1 {
              n181 = Index Array(array=w692, index=w691) -> (element=w690:dbl)
              n182 = global read "GVaktuelleTDMS.vi" "aktuelleTDMS-DateiECD2"() -> (w688:refnum<k34>)
              n183 = TDMS Read(0:w688, 7:"ECD2", 12:dbl[] []) -> (10:w693:dbl[])  [unwired: 4 in, 5 out]
              n184 = Array Size(array=w693) -> (size(s)=w695:i32)
              n185 = for {
                N: w695 -> [_]
                tunnel: [w698] -> w694 mode=indexing
                i -> [w701]
                n186 = To Double Precision Float(number=w701) -> (double precision float=w700:dbl)
                n187 = Divide(x=w700, y=10.0) -> (x/y=w698:dbl)
              }
              n188 = Bundle(w694, w693) -> (w689:cluster{dbl[], dbl[]})  [unwired: 1 in]
            }
          }
          n189 = global read "GVZeitenZyklen.vi" "Big Ben, Methodenzeit, Zykluszeit0, Zykluszeit1, Zykluszeit2A, Zykluszeit2B"() -> (w636:dbl[])
          "Big Ben, Methodenzeit, Zykluszeit0, Zykluszeit1, Zykluszeit2A, Zykluszeit2B" <- w636
          n190 = global read "GVMethodenwechsel.vi" "Methodenwechsel?"() -> (w669:bool)
          n191 = local read "veränderte Methode benutzen"() -> (w668:bool)
          n192 = global read "gvbooleschRT.vi" "global stop RT"() -> (w670:bool)
          n193 = global read "GVZeitenZyklen.vi" "ZyklusNummern"() -> (w635:i32[])
          "ZyklusNummern" <- w635
          n194 = Or(x=w669, y=w670) -> (x .or. y?=w672:bool)
          n195 = Or(x=w672, y=w668) -> (x .or. y?=w671:bool)
          n196 = Subtract(x="HK1YMax", y="HK1YMin") -> (x-y=w649:dbl)
          n197 = Subtract(x="HK2YMax", y="HK2YMin") -> (x-y=w644:dbl)
          n198 = call "AnzeigeGV.vi"("veränderte Methode benutzen"=w668, "Zykluslängen [s]"=w632, "Cluster1"=w667, "Big Ben, Methodenzeit, Zykluszeit0, Zykluszeit1, Zykluszeit2A, Zykluszeit2B"=w636, "Zyklusnummern 0, 1, 2A, 2B"=w635, "Cluster2"=w666, "AnzeigeEinstellungen"=w665, "dargestellte Größe 1"="dargestellte Größe 1", "Zeitachse1"="Zeitachse1", "dargestellte Größe 2"="dargestellte Größe 2", "Zeitachse2"="Zeitachse2") -> ("Anzeige2"=→"Housekeeping2":cluster{dbl[], dbl[]}, "Cluster1"=w660:cluster{dbl[], dbl[], dbl[], dbl[]}, "x1Inkr"=w655:dbl, "Cluster2"=w659:cluster{dbl[], dbl[], dbl[], dbl[]}, "Anzeige1"=→"Housekeeping1":cluster{dbl[], dbl[]}, "AnzeigeEinstellungen"=w657:T7, "x2Max"=w654:dbl, "x2Inkr"=w653:dbl, "x1Max"=w652:dbl)  [unwired: 8 in]
          n199 = Divide(x=w649, y=10.0) -> (x/y=w647:dbl)
          n200 = Divide(x=w644, y=10.0) -> (x/y=w642:dbl)
          n201 = property on="Housekeeping1" class="XYGraph (strict)"("XScale.Minimum"=w633, "XScale.Maximum"=w654, "XScale.Increment"=w655, "YScale.Minimum"="HK1YMin", "YScale.Maximum"="HK1YMax", "YScale.Increment"=w647) -> ()  [unwired: 2 in, 2 out]
          n202 = property on="Housekeeping2" class="XYGraph (strict)"("XScale.Minimum"=w633, "XScale.Maximum"=w652, "XScale.Increment"=w653, "YScale.Minimum"="HK2YMin", "YScale.Maximum"="HK2YMax", "YScale.Increment"=w642) -> ()  [unwired: 2 in, 2 out]
          n203 = Subtract(x="DetYMax", y="DetYMin") -> (x-y=w639:dbl)
          n204 = global read "GVZeitenZyklen.vi" "ZyklusNummernGesamt"() -> (→"ZyklusNummernGesamt":i32[])
          n205 = Equal?(x=w628, y=w627) -> (x = y?=w625:bool)
          n206 = Divide(x=w630, y=20.0) -> (x/y=w631:dbl)
          n207 = Divide(x=w639, y=20.0) -> (x/y=w637:dbl)
          n208 = Equal?(x="Detektor", y=w620) -> (x = y?=w619:bool)
          n209 = Select(t=w623, s=w625, f=w624) -> (s? t:f=w618:cluster{dbl[], dbl[]})
          n210 = property on="Detektor" class="XYGraph (strict)"("XScale.Minimum"=w633, "XScale.Maximum"=w630, "XScale.Increment"=w631, "YScale.Minimum"="DetYMin", "YScale.Maximum"="DetYMax", "YScale.Increment"=w637) -> ()  [unwired: 2 in, 2 out]
          n211 = Select(t=w618, s=w619, f=cluster{dbl[], dbl[]} {[], []} ("s? t:f")) -> (s? t:f=w616:cluster{dbl[], dbl[]})
          n212 = Build Array(w622, w616) -> (→"Detektor":cluster{dbl[], dbl[]}[])
          n213 = call "Bis zum nächsten Vielfachen warten14"("Count(mSec)"=u32 1000) -> ()  [unwired: 1 out]
        }
        n214 = global read "GVZeitenZyklen.vi" "Big Ben, Methodenzeit, Zykluszeit0, Zykluszeit1, Zykluszeit2A, Zykluszeit2B"() -> (w407:dbl[])
        n215 = while "Zeit" {
          tunnel: w435 -> [w731]
          tunnel: [w726] -> w445
          tunnel: w450 -> [w730]
          tunnel: [w720] -> w444
          tunnel: w434 -> [w721]
          tunnel: w401 -> [w728]
          tunnel: w412 -> [w715]
          tunnel: [w712] -> w443
          i -> [w734]
          stop <- w717 stop-if-true
          n216 = Equal?(x=w734, y=0) -> (x = y?=w732:bool)
          n217 = And(x=w731, y=w732) -> (x .and. y?=w736:bool)
          n218 = xnode "Elapsed Timer"("reset"=w736) -> ("elapsed time (ms)"=w739:i32)  [unwired: 2 in, 1 out]
          n219 = global read "gvbooleschRT.vi" "global stop RT"() -> (w729:bool)
          n220 = global read "GVMethodenwechsel.vi" "Methodenwechsel?"() -> (w716:bool)
          n221 = local read "veränderte Methode benutzen"() -> (w719:bool)
          n222 = To Double Precision Float(number=w739) -> (double precision float=w738:dbl)
          n223 = Or(x=w716, y=w729) -> (x .or. y?=w718:bool)
          n224 = Divide(x=w738, y=1000.0) -> (x/y=w726:dbl)
          n225 = Or(x=w719, y=w718) -> (x .or. y?=w717:bool)
          n226 = Subtract(x=w726, y=w730) -> (x-y=w725:dbl)
          n227 = for {
            tunnel: w728 -> [w742] mode=indexing
            tunnel: w725 -> [w743]
            tunnel: [w741] -> w727 mode=indexing
            tunnel: [w740] -> w724 mode=indexing
            n228 = Quotient & Remainder(x=w743, y=w742) -> (x-y*floor(x/y)=w741:dbl, floor(x/y)=w740:dbl)
          }
          n229 = Build Array (concatenate)(w726, w725, w727) -> (w714:dbl[])
          n230 = global write "GVZeitenZyklen.vi" "Big Ben, Methodenzeit, Zykluszeit0, Zykluszeit1, Zykluszeit2A, Zykluszeit2B"(w714) -> ()
          n231 = To Long Integer(number=w724) -> (32bit integer=w713:i32[])
          n232 = global write "GVZeitenZyklen.vi" "ZyklusNummern"(w713) -> ()
          n233 = Add(x=w713, y=w715) -> (x+y=w712:i32[])
          n234 = Index Array(array=w713, index=1 ("Index")) -> (element=w722:i32)
          n235 = Add(x=w722, y=w721) -> (x+y=w720:i32)
          n236 = global write "GVZeitenZyklen.vi" "ZyklusNummernGesamt"(w712) -> ()
          n237 = call "Bis zum nächsten Vielfachen warten15"("Count(mSec)"=u32 50) -> ()  [unwired: 1 out]
        }
        n238 = Index Array(array=w407, index=3 ("Index")) -> (element=w405:dbl)
        n239 = while {
          tunnel: w455 -> [w482]
          tunnel: w454 -> [w481]
          tunnel: w370 -> [w496]
          shift-right: [w497] -> w446
          shift-left: w453 -> [w498]
          tunnel: w367 -> [w492]
          tunnel: w366 -> [w486]
          shift-right: [w483] -> _
          shift-left: w405 -> [w487]
          stop <- w499 stop-if-true
          n240 = global read "gvbooleschRT.vi" "global stop RT"() -> (w502:bool)
          n241 = local read "veränderte Methode benutzen"() -> (w500:bool)
          n242 = global read "GVMethodenwechsel.vi" "Methodenwechsel?"() -> (w501:bool)
          n243 = Compound Arithmetic op=OR(w502, w501, w500) -> (w499:bool)
          n244 = global read "GVZeitenZyklen.vi" "Big Ben, Methodenzeit, Zykluszeit0, Zykluszeit1, Zykluszeit2A, Zykluszeit2B"() -> (w494:dbl[])
          n245 = Index Array(array=w494, index=3 ("Index")) -> (element=w483:dbl)
          n246 = Greater Or Equal?(x=w483, y=w492) -> (x >= y?=w491:bool)
          n247 = Less?(x=w487, y=w492) -> (x < y?=w490:bool)
          n248 = Greater Or Equal?(x=w483, y=w486) -> (x >= y?=w489:bool)
          n249 = Less?(x=w487, y=w486) -> (x < y?=w488:bool)
          n250 = And(x=w489, y=w488) -> (x .and. y?=w485:bool)
          n251 = And(x=w491, y=w490) -> (x .and. y?=w480:bool)
          n252 = Or(x=w480, y=w485) -> (x .or. y?=w484:bool)
          n253 = And(x=w496, y=w484) -> (x .and. y?=w495:bool)
          n254 = case shown="True" w495 {
            tunnel: w498 -> [w504 w505]
            tunnel: [w504 w509] -> w497
            tunnel: w482 -> [_ w508]
            tunnel: w481 -> [_ w507]
            tunnel: w480 -> [_ w506]
            frame False {
            }
            frame True {
              n255 = call "MSDateienSchicken02-15.vi"("MSNummer"=w505, "MSa?"=w506, "Dateipfad:fromcriordy"=w507, "Dateipfad:fromcriocmd"=w508) -> ()  [unwired: 1 in]
              n256 = Increment(x=w505) -> (x+1=w509:i32)
            }
          }
          n257 = call "Bis zum nächsten Vielfachen warten13"("Count(mSec)"=u32 100 ("Zu wartende ms")) -> ()  [unwired: 1 out]
        }
        n258 = global read "gvbooleschRT.vi" "global stop RT"() -> (w461:bool)
      }
      n259 = while {
        tunnel: w252 -> [w353]
        stop <- w356 stop-if-true
        n260 = global read "GVZeitenZyklen.vi" "Big Ben, Methodenzeit, Zykluszeit0, Zykluszeit1, Zykluszeit2A, Zykluszeit2B"() -> (w344:dbl[])
        n261 = call "Bis zum nächsten Vielfachen warten2"("Count(mSec)"=u32 1000) -> ()  [unwired: 1 out]
        n262 = global read "GVZeitenZyklen.vi" "ZyklusNummernGesamt"() -> (w342:i32[])
        n263 = global read "GVHK1Hz.vi" "Mod1Mod2Mod3/AITrapsMachs1Hz"() -> (w348:dbl[])
        n264 = global read "GVZeitenZyklen.vi" "ZyklusNummern"() -> (w343:i32[])
        n265 = global read "GVProbenvol.vi" "Probenvol.1"() -> (w341:dbl)
        n266 = global read "GVProbenvol.vi" "Probenvol.2"() -> (w340:dbl)
        n267 = global read "GVaktuelleTDMS.vi" "aktuelleTDMS-DateiHK"() -> (w347:refnum<k34>)
        n268 = global read "GVMWHorst.vi" "MWHorst"() -> (w349:dbl[])
        n269 = Index Array(array=w342, index=1 ("Index")) -> (element=w345:i32)
        n270 = To Double Precision Float(number=w345) -> (double precision float=w351:dbl)
        n271 = To Double Precision Float(number=w343) -> (double precision float=w350:dbl[])
        n272 = global read "gvbooleschRT.vi" "global stop RT"() -> (w356:bool)
        n273 = Build Array (concatenate)(w351, w350, w344, w348, w349, w341, w340) -> (w352:dbl[])
        n274 = TDMS Write(0:w347, 1:enum16{"decimated", "interleaved"}."interleaved" ("Daten-Layout (0:dezimiert)"), 7:w353, 9:w352) -> ()  [unwired: 2 in, 4 out]
      }
      n275 = while {
        stop <- w260 stop-if-true
        n276 = global read "GVECDs.vi" "ECD1Empfangen?"() -> (w258:bool)
        n277 = global read "GVECDs.vi" "ECD2Empfangen?"() -> (w257:bool)
        n278 = call "Bis zum nächsten Vielfachen warten3"("Count(mSec)"=u32 100) -> ()  [unwired: 1 out]
        n279 = case shown="True" w258 {
          frame False {
          }
          frame True {
            n280 = global read "GVaktuelleTDMS.vi" "aktuelleTDMS-DateiECD1"() -> (w268:refnum<k34>)
            n281 = global write "GVECDs.vi" "ECD1Empfangen?"(FALSE ("ECD1Empfangen?")) -> ()
            n282 = global read "GVECDs.vi" "ECD1MW"() -> (w267:dbl[])
            n283 = TDMS Write(0:w268, 7:"ECD1", 9:w267) -> ()  [unwired: 3 in, 4 out]
          }
        }
        n284 = case shown="True" w257 {
          frame False {
          }
          frame True {
            n285 = global read "GVaktuelleTDMS.vi" "aktuelleTDMS-DateiECD2"() -> (w264:refnum<k34>)
            n286 = global write "GVECDs.vi" "ECD2Empfangen?"(FALSE ("ECD2Empfangen?")) -> ()
            n287 = global read "GVECDs.vi" "ECD2MW"() -> (w263:dbl[])
            n288 = TDMS Write(0:w264, 7:"ECD2", 9:w263) -> ()  [unwired: 3 in, 4 out]
          }
        }
        n289 = global read "gvbooleschRT.vi" "global stop RT"() -> (w260:bool)
      }
      n290 = Index Array(array=w166, index #1=0 ("Index"), index #2=1 ("Index"), index #3=2 ("Index"), index #4=3 ("Index")) -> (element #1=w212:i32, element #2=w211:i32, element #3=w214:i32, element #4=w213:i32)
      n291 = Add(x=w214, y=w213) -> (x+y=w210:i32)
      n292 = Build Array(w212, w211, w210) -> (w209:i32[])
      n293 = for {
        N: 1 -> [_]
        tunnel: w171 -> [w338]
        tunnel: [w338] -> w203
        n294 = call "Warten8"("Count(mSec)"=u32 100) -> ()  [unwired: 1 out]
      }
      n295 = Index Array(array=w209, index #1=0 ("Index"), index #2=1 ("Index")) -> (element #1=w231:i32, element #2=w229:i32)
      n296 = Split 1D Array(array=w206, index=w231) -> (first subarray=w238:string[], second subarray=w240:string[])
      n297 = Split 1D Array(array=w208, index=w231) -> (first subarray=w235:dbl[], second subarray=w239:dbl[])
      n298 = Split 1D Array(array=w207, index=w231) -> (first subarray=w228:string[], second subarray=w230:string[])
      n299 = Concatenate Strings("?SE0,GDATA" ("Schreibpuffer"), "\r") -> (w178:string)
      n300 = Add Array Elements(numeric array=w209) -> (sum=w219:i32)
      n301 = Split 1D Array(array=w239, index=w229) -> (first subarray=w234:dbl[], second subarray=w233:dbl[])
      n302 = Split 1D Array(array=w240, index=w229) -> (first subarray=w237:string[], second subarray=w236:string[])
      n303 = Split 1D Array(array=w230, index=w229) -> (first subarray=w227:string[], second subarray=w226:string[])
      n304 = global read "GVVentilposition.vi" "Ventilposition"() -> (w177:i32)
      n305 = Bundle(w238, w237, w236, w235, w234, w233) -> (w232:T20)  [unwired: 1 in]
      n306 = Bundle(w228, w227, w226, w178, w178) -> (w225:T21)  [unwired: 1 in]
      n307 = Bundle(w222, w222, w222) -> (w221:cluster{string[], string[], string[]})  [unwired: 1 in]
      n308 = Initialize Array(-1.0 ("Element"), w219) -> (w204:dbl[])
      n309 = Bundle(w224, w224, w224) -> (w223:cluster{i32, i32, i32})  [unwired: 1 in]
      n310 = while {
        shift-right: [w324] -> _
        shift-left: bool[] [TRUE, TRUE, TRUE, TRUE, TRUE, TRUE] -> [w313]
        shift-right: [w303] -> _
        shift-left: w204 -> [w317]
        tunnel: w203 -> [w302]
        shift-right: [w322] -> _
        shift-left: string[] ["", "", "", "", "", ""] -> [w323]
        shift-right: [w304] -> _
        shift-left: w204 -> [w321]
        tunnel: w205 -> [w320]
        tunnel: w208 -> [w319]
        shift-right: [w306] -> _
        shift-left: w221 -> [w308]
        tunnel: w231 -> [w315]
        tunnel: w229 -> [w316]
        tunnel: w232 -> [w318]
        tunnel: w225 -> [w311]
        shift-right: [w310] -> _
        shift-left: w223 -> [w312]
        shift-right: [w299] -> _
        shift-left: w177 -> [w301]
        stop <- w305 stop-if-true
        n311 = global read "GVHorstSP.vi" "HorstSP"() -> (w303:dbl[])
        n312 = Not Equal?(x=w303, y=w317) -> (x != y?=w309:bool)
        n313 = call "NeueSP.vi"("Anzahl2"=w316, "Anzahl1"=w315, "AlteSP"=w317, 7:"NeueSP"=w303, "BefehleCluster"=w308, 10:"NeueSP"=w309, "ClusterFest"=w318) -> ("BefehleCluster"=w307:T22)  [unwired: 4 in]
        n314 = call "MPVSenden.vi"("Ventilposition"=w301, "FPGA VI Reference"=w302) -> ("Ventilposition"=w299:i32, "FPGA VI Reference"=w300:refnum<k20>)
        n315 = call "Senden.vi"("FPGA VI Reference In"=w300, "BefehlsCluster"=w307, "Senden?"=w313, "Abfragenr.Cluster"=w312, "AbfragenCluster"=w311) -> ("Senden?"=w314:bool[], "Abfragenr.Cluster"=w310:cluster{i32, i32, i32}, "BefehlsCluster"=w306:T22)  [unwired: 1 in]
        n316 = call "SeriellRead.vi"("SkalierungsfaktorHorst"=w319, "VorwortHorst"=w320, 8:w321, "Zwischenspeicher"=w323, "Senden?"=w314, "FPGA VI Reference In"=w300) -> ("Senden?"=w324:bool[], "Zwischenspeicher"=w322:string[], 3:w304)  [unwired: 3 in]
        n317 = global read "gvbooleschRT.vi" "global stop RT"() -> (w305:bool)
        n318 = global write "GVMWHorst.vi" "MWHorst"(w304) -> ()
      }
      n319 = Unbundle(w197) -> ("Dateiordner Housekeeping"=w196:path, "DateiordnerECD1"=w194:path, "DateiordnerECD2"=w193:path, "Dateiname Housekeeping"=w195:string, "DateinameECD1"=w192:string, "DateinameECD2"=w191:string, "tdms0"=w190:refnum<k34>, "tdms1"=w189:refnum<k34>, "tdms0"=w188:refnum<k34>, "tdms1"=w187:refnum<k34>, "tdms0"=w186:refnum<k34>, "tdms1"=w185:refnum<k34>)
      n320 = while {
        shift-right: [w278] -> w182
        shift-left: w186 -> [w270]
        shift-right: [w279] -> w181
        shift-left: w185 -> [w272]
        shift-right: [w276] -> _
        shift-left: w198 -> [w280]
        tunnel: w193 -> [w275]
        tunnel: w191 -> [w274]
        stop <- w282 stop-if-true
        n321 = global read "GVZeitenZyklen.vi" "ZyklusNummernGesamt"() -> (w269:i32[])
        n322 = call "Bis zum nächsten Vielfachen warten6"("Count(mSec)"=u32 500) -> ()  [unwired: 1 out]
        n323 = Index Array(array=w269, index=3 ("Index")) -> (element=w276:i32)
        n324 = Greater?(x=w276, y=w280) -> (0:w273:bool)
        n325 = Select(t=w272, s=w273, f=w270) -> (s? t:f=w271:refnum<k34>)
        n326 = global write "GVaktuelleTDMS.vi" "aktuelleTDMS-DateiECD2"(w271) -> ()
        n327 = local read "Methode"() -> (w277:i32)
        n328 = global read "gvbooleschRT.vi" "global stop RT"() -> (w282:bool)
        n329 = call "AktuelleTDMS.vi"("AktuelleTDMS"=w270, "Dateiordner"=w275, "NächsteTDMS"=w272, "NeuerZyklus?"=w273, "Methodennummer"=w277, "Zyklnumges"=w276, "Dateiname"=w274) -> ("AktuelleTDMS"=w278:refnum<k34>, "NächsteTDMS"=w279:refnum<k34>)  [unwired: 5 in, 2 out]
      }
      n330 = while {
        shift-right: [w846] -> w255
        shift-left: w190 -> [w840]
        shift-right: [w850] -> w254
        shift-left: w189 -> [w842]
        shift-right: [w844] -> _
        shift-left: w198 -> [w851]
        tunnel: w195 -> [w847]
        tunnel: w196 -> [w848]
        stop <- w853 stop-if-true
        n331 = global read "GVZeitenZyklen.vi" "ZyklusNummernGesamt"() -> (w839:i32[])
        n332 = call "Bis zum nächsten Vielfachen warten5"("Count(mSec)"=u32 500) -> ()  [unwired: 1 out]
        n333 = Index Array(array=w839, index=1 ("Index")) -> (element=w844:i32)
        n334 = Greater?(x=w844, y=w851) -> (0:w843:bool)
        n335 = Select(t=w842, s=w843, f=w840) -> (s? t:f=w841:refnum<k34>)
        n336 = global write "GVaktuelleTDMS.vi" "aktuelleTDMS-DateiHK"(w841) -> ()
        n337 = local read "Methode"() -> (w849:i32)
        n338 = global read "gvbooleschRT.vi" "global stop RT"() -> (w853:bool)
        n339 = call "AktuelleTDMS.vi"("AktuelleTDMS"=w840, "Dateiordner"=w848, "NächsteTDMS"=w842, "NeuerZyklus?"=w843, "Methodennummer"=w849, "Zyklnumges"=w844, "Dateiname"=w847) -> ("AktuelleTDMS"=w846:refnum<k34>, "NächsteTDMS"=w850:refnum<k34>)  [unwired: 5 in, 2 out]
      }
      n340 = while {
        shift-right: [w293] -> w184
        shift-left: w188 -> [w285]
        shift-right: [w294] -> w183
        shift-left: w187 -> [w287]
        shift-right: [w291] -> _
        shift-left: w198 -> [w295]
        tunnel: w194 -> [w290]
        tunnel: w192 -> [w289]
        stop <- w297 stop-if-true
        n341 = global read "GVZeitenZyklen.vi" "ZyklusNummernGesamt"() -> (w284:i32[])
        n342 = call "Bis zum nächsten Vielfachen warten4"("Count(mSec)"=u32 500) -> ()  [unwired: 1 out]
        n343 = Index Array(array=w284, index=2 ("Index")) -> (element=w291:i32)
        n344 = Greater?(x=w291, y=w295) -> (0:w288:bool)
        n345 = Select(t=w287, s=w288, f=w285) -> (s? t:f=w286:refnum<k34>)
        n346 = global write "GVaktuelleTDMS.vi" "aktuelleTDMS-DateiECD1"(w286) -> ()
        n347 = local read "Methode"() -> (w292:i32)
        n348 = global read "gvbooleschRT.vi" "global stop RT"() -> (w297:bool)
        n349 = call "AktuelleTDMS.vi"("AktuelleTDMS"=w285, "Dateiordner"=w290, "NächsteTDMS"=w287, "NeuerZyklus?"=w288, "Methodennummer"=w292, "Zyklnumges"=w291, "Dateiname"=w289) -> ("AktuelleTDMS"=w293:refnum<k34>, "NächsteTDMS"=w294:refnum<k34>)  [unwired: 5 in, 2 out]
      }
    }
    frame #2 {
      n350 = TDMS Close(11:w867) -> ()  [unwired: 1 in, 2 out]
      n351 = TDMS Close(11:w866) -> ()  [unwired: 1 in, 2 out]
      n352 = TDMS Close(11:w862) -> ()  [unwired: 1 in, 2 out]
      n353 = TDMS Close(11:w861) -> ()  [unwired: 1 in, 2 out]
      n354 = TDMS Close(11:w860) -> ()  [unwired: 1 in, 2 out]
      n355 = TDMS Close(11:w859) -> ()  [unwired: 1 in, 2 out]
      n356 = xnode "Read/Write Control"("FPGA VI Reference In"=w865, "global stop"=TRUE) -> ("FPGA VI Reference Out"=w864:refnum<k20>)  [unwired: 1 in, 1 out]
      n357 = xnode "Close FPGA VI Reference"("FPGA VI Reference In"=w864) -> ()  [unwired: 1 in, 1 out]
    }
  }
  n358 = Open/Create/Replace File(file path (use dialog)=path "c:/methoden.per" ("Datei (Dialog verwenden)"), operation (0:open)=T3."open" ("Operation (0:Öffnen)")) -> (refnum out=w6:refnum<file>)  [unwired: 4 in, 2 out]
  n359 = Read from Binary File(5:T1 [] ("Methoden"), 11:w6) -> (2:w3:T1, 3:w5:refnum<file>)  [unwired: 4 in, 2 out]
  n360 = Close File(refnum=w5) -> ()  [unwired: 1 in, 2 out]
